vi "Main.vi"() -> ()   [LabVIEW 2019]
uses:
  SubVi/TypeDefs/ModeControl.ctl
  SubVi/TypeDefs/MotorDataControl.ctl
  SubVi/TypeDefs/PerturbationControl.ctl
  SubVi/TypeDefs/GameMode.ctl
  <vilib>/myRIO/Instrument Drivers/Onboard IO/AO/typedefs/AO Reference.ctl
  <vilib>/myRIO/Common/Instrument Driver Framework/Utilities/typedefs/myRIO Generic Hardware Reference.ctl
  <vilib>/myRIO/Common/Instrument Driver Framework/Utilities/typedefs/Hardware Version Enum.ctl
  <vilib>/myRIO/Common/Instrument Driver Framework/Utilities/typedefs/myRIO v1.0 Reference.ctl
  <vilib>/myRIO/Common/Instrument Driver Framework/Utilities/typedefs/Generic FPGA Reference.ctl
  <vilib>/myRIO/Common/Instrument Driver Framework/myRIO v1.0/AO/typedefs/AO Channels List.ctl
  <vilib>/myRIO/Common/Instrument Driver Framework/myRIO v1.0/AO/typedefs/AO Channels Enum.ctl
  <vilib>/myRIO/Common/Instrument Driver Framework/Utilities/typedefs/Analog Scaling Constants List.ctl
  <vilib>/myRIO/Common/Instrument Driver Framework/Utilities/typedefs/Analog Scaling Constants.ctl
  <vilib>/userDefined/High Color/nirio_resource_hc.ctl
  <vilib>/myRIO/Instrument Drivers/Onboard IO/DIO/typedefs/DIO Reference.ctl
  <vilib>/myRIO/Common/Instrument Driver Framework/myRIO v1.0/DIO/typedefs/DIO Channels List.ctl
  <vilib>/myRIO/Common/Instrument Driver Framework/myRIO v1.0/DIO/typedefs/DIO Channels Enum.ctl
  Tutorial/Shared VIs/TypeDef_TDMS_States.ctl
  <vilib>/Platform/TimedLoop/XDataNode/timing_clust.ctl
  <vilib>/Platform/TimedLoop/XDataNode/nitl_modes.ctl
  <vilib>/Platform/TimedLoop/XDataNode/wakeup.ctl
  SubVi/TypeDefs/PositionDataControl.ctl
  <vilib>/myRIO/Common/Instrument Driver Framework/myRIO v1.0/Encoder/typedefs/Encoder Signal Mode.ctl
  <vilib>/myRIO/Instrument Drivers/Onboard IO/Encoder/typedefs/Encoder Reference.ctl
  <vilib>/myRIO/Common/Instrument Driver Framework/myRIO v1.0/Encoder/typedefs/Encoder Channels Enum.ctl
  <vilib>/myRIO/Common/Instrument Driver Framework/myRIO v1.0/Encoder/typedefs/Encoder Configuration v1.0.ctl
  <vilib>/myRIO/Instrument Drivers/Onboard IO/AI/typedefs/AI Reference.ctl
  <vilib>/myRIO/Common/Instrument Driver Framework/myRIO v1.0/AI/typedefs/AI Channels List.ctl
  <vilib>/myRIO/Common/Instrument Driver Framework/myRIO v1.0/AI/typedefs/AI Channels Enum.ctl
  <vilib>/myRIO/Common/Instrument Driver Framework/Utilities/vis/Is FPGA Ref Available.vi
  <vilib>/myRIO/Common/Instrument Driver Framework/myRIO v1.0/AO/vis/myRIO v1.1 Open AO.vi
  <vilib>/myRIO/Instrument Drivers/Onboard IO/AO/vis/Write.vi
  <vilib>/myRIO/Common/Instrument Driver Framework/myRIO v1.0/DIO/vis/myRIO v1.1 Open DIO.vi
  <vilib>/myRIO/Instrument Drivers/Onboard IO/DIO/vis/Write.vi
  <vilib>/myRIO/Common/Instrument Driver Framework/myRIO v1.0/AI/vis/myRIO v1.1 Open AI.vi
  <vilib>/myRIO/Instrument Drivers/Onboard IO/AI/vis/Read.vi
  <vilib>/myRIO/Common/Instrument Driver Framework/myRIO v1.0/Encoder/vis/myRIO v1.1 Open Encoder.vi
  <vilib>/myRIO/Instrument Drivers/Onboard IO/Encoder/vis/Read.vi
  <vilib>/myRIO/Common/Instrument Driver Framework/Utilities/vis/Validate Channels.vi
  <vilib>/myRIO/Common/Instrument Driver Framework/myRIO v1.0/AO/vis/myRIO v1.0 Reserve AO.vi
  <vilib>/myRIO/Common/Instrument Driver Framework/myRIO v1.0/DIO/vis/myRIO v1.0 Reserve DIO.vi
  <vilib>/myRIO/Common/Instrument Driver Framework/myRIO v1.0/AI/vis/myRIO v1.0 Reserve AI.vi
  <vilib>/myRIO/Common/Instrument Driver Framework/myRIO v1.0/Encoder/vis/myRIO v1.0 Reserve Encoder.vi
  <vilib>/myRIO/Common/Instrument Driver Framework/myRIO v1.0/AO/vis/myRIO v1.0 Build MUX Configuration AO.vi
  <vilib>/myRIO/Common/Instrument Driver Framework/myRIO v1.0/Resource Manager/vis/myRIO v1.0 Reserve Channel List.vi
  <vilib>/myRIO/Common/Instrument Driver Framework/myRIO v1.0/DIO/vis/myRIO v1.0 Build MUX Configuration DIO.vi
  <vilib>/myRIO/Common/Instrument Driver Framework/myRIO v1.0/AI/vis/myRIO v1.0 Build MUX Configuration AI.vi
  <vilib>/myRIO/Common/Instrument Driver Framework/myRIO v1.0/Encoder/vis/myRIO v1.0 Build MUX Configuration Encoder.vi
  <vilib>/myRIO/Common/Instrument Driver Framework/myRIO v1.0/Resource Manager/vis/myRIO v1.0 Reserve Channel.vi
  <vilib>/myRIO/Common/Instrument Driver Framework/myRIO v1.0/Resource Manager/vis/myRIO v1.0 Unreserve Channel.vi
  <vilib>/myRIO/Common/Instrument Driver Framework/myRIO v1.0/Resource Manager/vis/myRIO v1.0 Create Configuration List.vi
  <vilib>/myRIO/Common/Instrument Driver Framework/myRIO v1.0/Resource Manager/vis/myRIO v1.0 Build Mutex Name.vi
  <vilib>/Utility/VariantDataType/GetNumericInfo.vi
  <vilib>/Utility/error.llb/Error Cluster From Error Code.vi
  <vilib>/myRIO/Common/Instrument Driver Framework/myRIO v1.0/myRIO v1.1 Open.vi
  <vilib>/myRIO/Common/Instrument Driver Framework/myRIO v1.0/AO/vis/myRIO v1.0 Get Scaling Constants AO.vi
  <vilib>/myRIO/Common/Instrument Driver Framework/Utilities/vis/IO Manager.vi
  <vilib>/myRIO/Common/Instrument Driver Framework/Utilities/vis/Configuration Manager.vi
  <vilib>/myRIO/Common/Instrument Driver Framework/myRIO v1.0/myRIO v1.0 Close.vi
  <vilib>/myRIO/Common/Instrument Driver Framework/myRIO v1.0/AO/vis/myRIO v1.0 Write AO.vi
  <vilib>/myRIO/Common/Instrument Driver Framework/myRIO v1.0/Resource Manager/vis/myRIO v1.0 Configure IO.vi
  <vilib>/myRIO/Common/Instrument Driver Framework/myRIO v1.0/DIO/vis/myRIO v1.0 Write DIO.vi
  <vilib>/myRIO/Common/Instrument Driver Framework/myRIO v1.0/Encoder/vis/myRIO v1.0 Configure Encoder.vi
  <vilib>/myRIO/Common/Instrument Driver Framework/myRIO v1.0/Encoder/vis/myRIO v1.0 Read Encoder.vi
  <vilib>/myRIO/Common/Instrument Driver Framework/myRIO v1.0/AI/vis/myRIO v1.0 Get Scaling Constants AI.vi
  <vilib>/myRIO/Common/Instrument Driver Framework/myRIO v1.0/AI/vis/myRIO v1.0 Read AI.vi
  <vilib>/addons/control/pid/pid.llb/PID (DBL).vi
  <vilib>/myRIO/Express VI/Onboard IO/AO/AO Express VI.xnode
  <vilib>/myRIO/Instrument Drivers/Onboard IO/AO/vis/myRIO AO Open.xnode
  <vilib>/myRIO/Express VI/Onboard IO/DO/DO Express VI.xnode
  <vilib>/myRIO/Instrument Drivers/Onboard IO/DIO/vis/myRIO DIO Open.xnode
  <vilib>/Platform/TimedLoop/XDataNode/XDataNode.xnode
  <vilib>/myRIO/Express VI/Onboard IO/Encoder/Encoder Express VI.xnode
  <vilib>/myRIO/Instrument Drivers/Onboard IO/Encoder/vis/myRIO Encoder Open.xnode
  <vilib>/myRIO/Common/Instrument Driver Framework/myRIO v1.0/Encoder/typedefs/Encoder Count Direction Enum.ctl
  <vilib>/myRIO/Express VI/Onboard IO/AI/AI Express VI.xnode
  <vilib>/myRIO/Instrument Drivers/Onboard IO/AI/vis/myRIO AI Open.xnode
  <vilib>/Platform/TimedLoop/XDataNode/XDNodeRunTimeDep.lvlib
  <vilib>/addons/control/pid/NI_PID_pid.lvlib
  <vilib>/myRIO/Instrument Drivers/Onboard IO/AO/AO.lvlib
  <vilib>/myRIO/Instrument Drivers/Onboard IO/DIO/DIO.lvlib
  <vilib>/myRIO/Instrument Drivers/Onboard IO/Encoder/Encoder.lvlib
  <vilib>/myRIO/Instrument Drivers/Onboard IO/AI/AI.lvlib
panel:
  out "LinPot mm (center to finger) 2":dbl
  out "LinPot mm (center to finger)":dbl
  out "Right Poti Offset":dbl
  out "Left Poti Offset":dbl
  out "Right Poti Gradient":dbl
  out "Left Poti Gradient":dbl
  out "LX gradient":dbl
  out "LY gradient":dbl
  out "RY gradient":dbl
  out "RX gradient":dbl
  out "Safety Warning":bool
  out "Safety Been Triggered":bool
  out "TimeStampData":cluster{"time":string}
  out "UDPTimestamp":T1
  out "Force Sensor Faulty":bool
  out "Pots Faulty":bool
  out "ForceBiasGR_R":dbl
  out "ForceBiasPS_R":dbl
  out "Left F_y[N]":dbl(graph)
  out "Left F_x[N]":dbl(graph)
  out "define_dX_GR":bool
  out "Applied Torque Rotation":dbl(graph)
  out "PS Setpoint/ProcessVar [mm]":T2(graph) caption="Response"
  out "dtheta PS (deg)":dbl
  out "GR Setpoint/ProcessVar [mm]":T2(graph) caption="Response"
  out "dx GR (mm)":dbl
  out "Potentiometers_array":dbl[](array[numeric])
  out "PID output voltage rotation":dbl(graph)
  out "PID output voltage translation":dbl(graph)
  out "ForceBiasGR_L":dbl
  out "ForceBiasPS_L":dbl
  out "NewPerturbation":bool
  out "JSON string":string
  out "Baseline[N]":dbl
  out "Reached":bool
  out "ForcePeak[N]":dbl
  out "ForceTransBuffer[N]":ext[](array[numeric])
  out "Game":T4
  out "UDPPerturbation":T5
  out "Perturbation":T6
  out "MotorData":T7
  out "UDPGame":T5
  in  "SaveData (Manual)":bool
  out "Main Loop Time":i32
  out "Perturbation Response":cluster{"PositionTranslation":dbl, "Step":dbl}(graph) caption="Response"
  out "Target Position Rotation":dbl format="%#_13g"
  out "Target Position Translation":dbl format="%#_13g"
  out "Relative Pos Trans Saved":dbl format="%#_13g"
  out "Save Data":bool=TRUE
  out "isaved":i32
  out "Case":i32
  out "UDPSafety":T5
  out "InitialTranslation":dbl
  out "InitialRotation":dbl
  out "HardSafety":bool
  out "SoftSafety":bool
  out "AppliedTorqueRotation [Nmm]":dbl
  out "AbsolutePositionRotation":dbl
  out "AbsolutePositionTranslation":dbl
  out "AppliedForceRotation [N]":dbl
  out "AppliedForceTranslation [N]":dbl
  out "Right F_y[N]":dbl(graph)
  out "Right F_x[N]":dbl(graph)
  out "Finalize":bool
  out "VoltageTranslation":dbl
  out "VoltageRotation":dbl
  out "Calibration":T8
  out "Mode":T9
  out "MotorValues":T10
  out "UDPMotorValues":T5
  out "VelocityRotation":dbl
  out "VelocityTranslation":dbl
  out "CalibratorTranslation":dbl
  out "CalibratorRotation":dbl
  out "Period":i32
  out "LoopTime":dbl
  out "RelativePositionRotation":dbl
  out "RelativePositionTranslation":dbl
  out "UDPCalibration":T5
  out "UDPMotorData":T5
  out "UDPMode":T5
  out "IPAddress":i64
  out "UDPConnection":T5
  # "HELLO UPDATE"
  # "Green if data saving in progress"
  # "Force manual data save when pressed"
  # "To Giorgia:\nremember first to set \nthis index to 0 if you\nwant to control the\npronosupination DOF\nor to 1 if you want to\ncontrol the grasping\n\nAlways remember \nto set the stopPosition\n(for stop mode), \nor position&velocity (for\nmove mode) in a way that\nis feasible for the \nRelativePosition in which\nyou are. Do that ALWAYS \n1) before changing motorMode\n2) before changing \nMode from Wait to Run"
  # "Perturbation response in grasping"
  # "Green ON = no safety stop\nSoft = max force/pos/vel exceeded\nHard= sensor problem"
  # "Green ON = closing Labview \n(on Hard Safety or\nquit GUI/patient selection)"
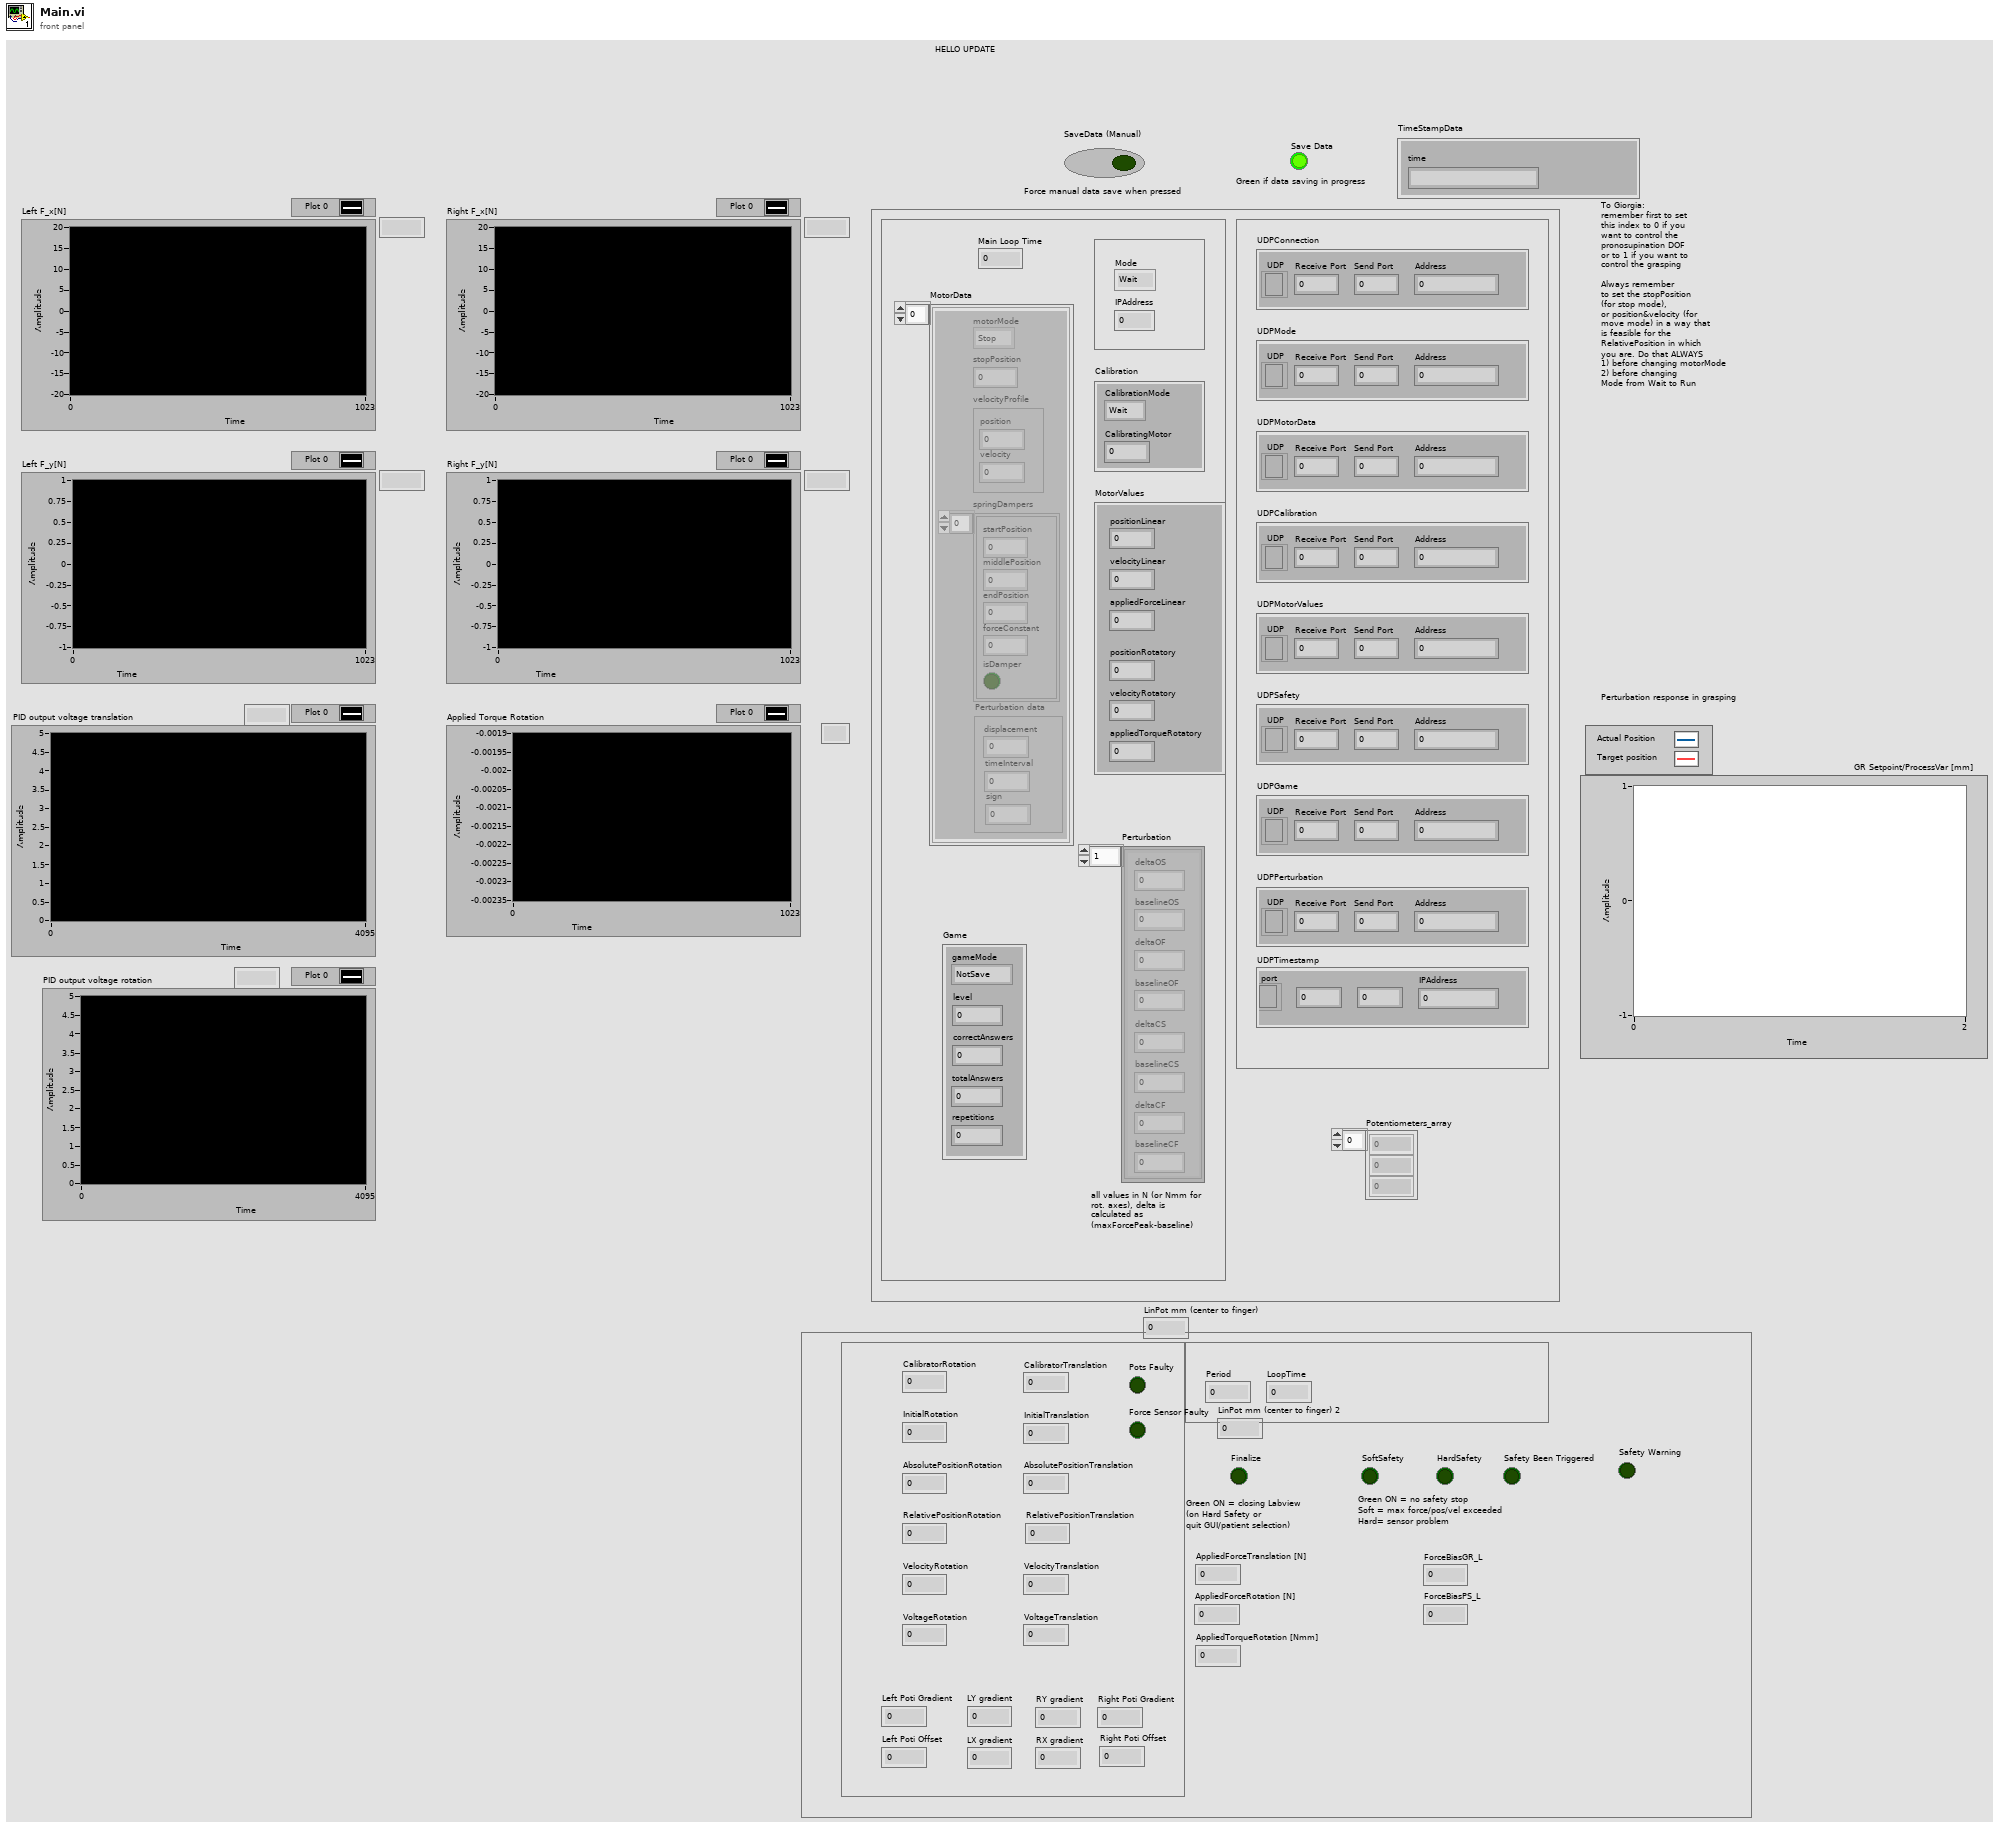
[diagram p1: front panel]
types:
  T1 = cluster{"port":refnum<k16>, i32, i32, "IPAddress":i64}
  T2 = cluster{"AbsolutePositionTranslation":dbl, "inverse delta GR":dbl}
  T3 = typedef "GameMode.ctl" = enum16{"NotSave", "Calibrate", "Training", "Test", "Summary"}
  T4 = cluster{"gameMode":T3, "level":dbl, "correctAnswers":dbl, "totalAnswers":dbl, "repetitions":dbl}
  T5 = cluster{"UDP":refnum<k16>, "Receive Port":i32, "Send Port":i32, "Address":i64}
  T6 = typedef "PerturbationControl.ctl" = cluster{"deltaOS":dbl, "baselineOS":dbl, "deltaOF":dbl, "baselineOF":dbl, "deltaCS":dbl, "baselineCS":dbl, "deltaCF":dbl, "baselineCF":dbl}[]
  T7 = typedef "MotorDataControl.ctl" = cluster{"motorMode":enum16{"Stop", "Move", "Force", "Perturbation"}, "stopPosition":dbl, "velocityProfile":cluster{"position":dbl, "velocity":dbl}, "springDampers":cluster{"startPosition":dbl, "middlePosition":dbl, "endPosition":dbl, "forceConstant":dbl, "isDamper":bool}[], "Perturbation data ":cluster{"displacement":dbl, "timeInterval":dbl, "sign":i64}}[]
  T8 = cluster{"CalibrationMode":enum16{"Wait", "Calibrate"}, "CalibratingMotor":i8}
  T9 = typedef "ModeControl.ctl" = enum16{"Wait", "Calibrate", "Run", "Safety", "Quit"}
  T10 = cluster{"positionLinear":dbl, "velocityLinear":dbl, "appliedForceLinear":dbl, "positionRotatory":dbl, "velocityRotatory":dbl, "appliedTorqueRotatory":dbl}
  T11 = typedef "AO.lvlib/AO Reference.ctl" = cluster{"myRIO Reference":T12, "AO Channel List":T16, "AO Scaling Constant List":T18}
  T12 = typedef "myRIO Generic Hardware Reference.ctl" = cluster{"myRIO Model":T13, "myRIO Hardware Reference":T14}
  T13 = typedef "Hardware Version Enum.ctl" = enum16{"Unknown", "myRIO-1900", "myRIO-1950", "roboRIO", "NI ELVIS RIO CM", "ELVIS III"}
  T14 = typedef "myRIO v1.0 Reference.ctl" = cluster{"Generic FPGA Reference":T15, "Allow multiple opens":bool}
  T15 = typedef "Generic FPGA Reference.ctl" = refnum<k20>
  T16 = typedef "AO Channels List.ctl" = T17[]
  T17 = typedef "AO Channels Enum.ctl" = enum16{"Not Connected", "AudioOut/Left", "AudioOut/Right", "C/AO0", "C/AO1", "A/AO0", "A/AO1", "B/AO0", "B/AO1"}
  T18 = typedef "Analog Scaling Constants List.ctl" = T19[]
  T19 = typedef "Analog Scaling Constants.ctl" = cluster{"LSB Weight (Volts)":dbl, "Offset (Volts)":dbl, "Signed?":bool}
  T20 = typedef "nirio_resource_hc.ctl" = tag
  T21 = typedef "DIO.lvlib/DIO Reference.ctl" = cluster{"myRIO Reference":T12, "DIO Channels List":T22}
  T22 = typedef "DIO Channels List.ctl" = T23[]
  T23 = typedef "DIO Channels Enum.ctl" = enum16{"Not Connected", "C/DIO0", "C/DIO1", "C/DIO2", "C/DIO3", "C/DIO4", "C/DIO5", "C/DIO6", "C/DIO7", "A/DIO0", "A/DIO1", "A/DIO2", "A/DIO3", "A/DIO4", "A/DIO5", "A/DIO6", "A/DIO7", "A/DIO8", "A/DIO9", "A/DIO10", "A/DIO11", "A/DIO12", "A/DIO13", "A/DIO14", "A/DIO15", "A/DIO16", "A/DIO17", "A/DIO18", "A/DIO19", "B/DIO0", "B/DIO1", "B/DIO2", "B/DIO3", "B/DIO4", "B/DIO5", "B/DIO6", "B/DIO7", "B/DIO8", "B/DIO9", "B/DIO10", "B/DIO11", "B/DIO12", "B/DIO13", "B/DIO14", "B/DIO15", "B/DIO16", "B/DIO17", "B/DIO18", "B/DIO19", "LED0", "LED1", "LED2", "LED3", "Button0", "DIO/DIO0", "DIO/DIO1", "DIO/DIO2", "DIO/DIO3", "DIO/DIO4", "DIO/DIO5", "DIO/DIO6", "DIO/DIO7", "DIO/DIO8", "DIO/DIO9", "SPI/CS0", "SPI/CS1", "SPI/CS2", "SPI/CS3", "LED RADIO (Green)", "LED RADIO (Red)", "LED COMM (Green)", "LED COMM (Red)", "LED MODE (Green)", "LED MODE (Red)"}
  T24 = typedef "TypeDef_TDMS_States.ctl" = enum16{"Do Nothing", "Create", "Write", "Close"}
  T25 = enum16{"open", "open or create", "create or replace", "create", "open (read-only)"}
  T26 = typedef "XDNodeRunTimeDep.lvlib/timing_clust.ctl" = cluster{"Expected End [f-1]":u64, "Actual End [f-1]":u64, "Finished Late? [f-1]":bool, "Expected End [i-1]":u64, "Actual End [i-1]":u64, "Finished Late? [i-1]":bool, "Expected Start [i]":u64, "Actual Start [i]":u64, "Expected Start [f]":u64, "Actual Start [f]":u64, "Source Name":string, "Structure Name":string, "Period":i64, "Deadline":i64, "Offset":i64, "Start":i64, "Priority":i32, "Timeout":i32, "Mode":T27, "Wakeup Reason":T28, "Error":errorcluster, "Source Type":string, "Secondary Source Type":string, "Global End Time":u64, "Global Start Time":u64, "Frame Duration":u64, "Iteration Duration":u64, "Assigned CPU":i32, "I/O Scan Engine Mode":u32}
  T27 = typedef "XDNodeRunTimeDep.lvlib/nitl_modes.ctl" = enum32{"No Change", "Process missed periods, maintain original phase", "Discard missed periods, maintain original phase", "Process missed periods, ignore original phase", "Discard missed periods, ignore original phase"}
  T28 = typedef "XDNodeRunTimeDep.lvlib/wakeup.ctl" = enum32{"Normal", "Aborted", "Asynchronous wakeup", "Timing source error", "Timed loop error", "Timeout"}
  T29 = typedef "PositionDataControl.ctl" = cluster{"Position":dbl, "Velocity":dbl}
  T30 = typedef "AI.lvlib/AI Reference.ctl" = cluster{"myRIO Reference":T12, "AI Channels List":T31, "AI Scaling Constants List":T18}
  T31 = typedef "AI Channels List.ctl" = T32[]
  T32 = typedef "AI Channels Enum.ctl" = enum16{"Not Connected", "AudioIn/Left", "AudioIn/Right", "C/AI0", "C/AI1", "A/AI0", "A/AI1", "A/AI2", "A/AI3", "A/AI4", "A/AI5", "A/AI6", "A/AI7", "B/AI0", "B/AI1", "B/AI2", "B/AI3", "B/AI4", "B/AI5", "B/AI6", "B/AI7", "AI/AI0", "AI/AI1", "AI/AI2", "AI/AI3", "A/AI0 (DIFF)", "A/AI1 (DIFF)", "A/AI2 (DIFF)", "A/AI3 (DIFF)", "B/AI0 (DIFF)", "B/AI1 (DIFF)", "B/AI2 (DIFF)", "B/AI3 (DIFF)"}
  T33 = typedef "Encoder.lvlib/Encoder Reference.ctl" = cluster{"myRIO Reference":T12, "Encoder Channels Enum":T34}
  T34 = typedef "Encoder Channels Enum.ctl" = enum16{"Not Connected", "C/ENC0", "C/ENC1", "A/ENC", "A/ENC0", "A/ENC1", "A/ENC2", "A/ENC3", "A/ENC4", "A/ENC5", "A/ENC6", "A/ENC7", "A/ENC8", "A/ENC9", "B/ENC", "B/ENC0", "B/ENC1", "B/ENC2", "B/ENC3", "B/ENC4", "B/ENC5", "B/ENC6", "B/ENC7", "B/ENC8", "B/ENC9", "DIO/ENC0", "DIO/ENC1", "DIO/ENC2", "DIO/ENC3", "DIO/ENC4"}
  T35 = typedef "Encoder Signal Mode.ctl" = enum16{"Quadrature phase signal", "Step and direction signal"}
  T36 = cluster{"startPosition":dbl, "middlePosition":dbl, "endPosition":dbl, "forceConstant":dbl, "isDamper":bool}[]
  T37 = cluster{"proportional gain (Kc)":dbl, "integral time (Ti, min)":dbl, "derivative time (Td, min)":dbl}
  T38 = cluster{"motorMode":enum16{"Stop", "Move", "Force", "Perturbation"}, "stopPosition":dbl, "velocityProfile":cluster{"position":dbl, "velocity":dbl}, "springDampers":cluster{"startPosition":dbl, "middlePosition":dbl, "endPosition":dbl, "forceConstant":dbl, "isDamper":bool}[], "Perturbation data ":cluster{"displacement":dbl, "timeInterval":dbl, "sign":i64}}
  T39 = cluster{"deltaOS":dbl, "baselineOS":dbl, "deltaOF":dbl, "baselineOF":dbl, "deltaCS":dbl, "baselineCS":dbl, "deltaCF":dbl, "baselineCF":dbl}
  T40 = cluster{"motorMode":enum16{"Stop", "Move", "Force", "Perturbation"}, "stopPosition":dbl, "velocityProfile":cluster{"position":dbl, "velocity":dbl}, "springDampers":cluster{"startPosition":dbl, "middlePosition":dbl, "endPosition":dbl, "forceConstant":dbl, "isDamper":bool}[], "Perturbation data ":cluster{"displacement":dbl, "timeInterval":dbl, "sign":i64}}[]
  T41 = cluster{"deltaOS":dbl, "baselineOS":dbl, "deltaOF":dbl, "baselineOF":dbl, "deltaCS":dbl, "baselineCS":dbl, "deltaCF":dbl, "baselineCF":dbl}[]
  T42 = cluster{"displacement":dbl, "timeInterval":dbl, "sign":i64}
  T43 = cluster{"RelativePositionTranslation":dbl, "dx GR (mm)":dbl}
  T44 = cluster{"RelativePositionTranslation":dbl, "RelativePositionTranslation":dbl}
  T45 = cluster{"RelativePositionRotation":dbl, "dtheta PS (deg)":dbl}
  T46 = cluster{"gameMode":i8, "level":dbl, "correctAnswers":dbl, "totalAnswers":dbl, "repetitions":dbl}
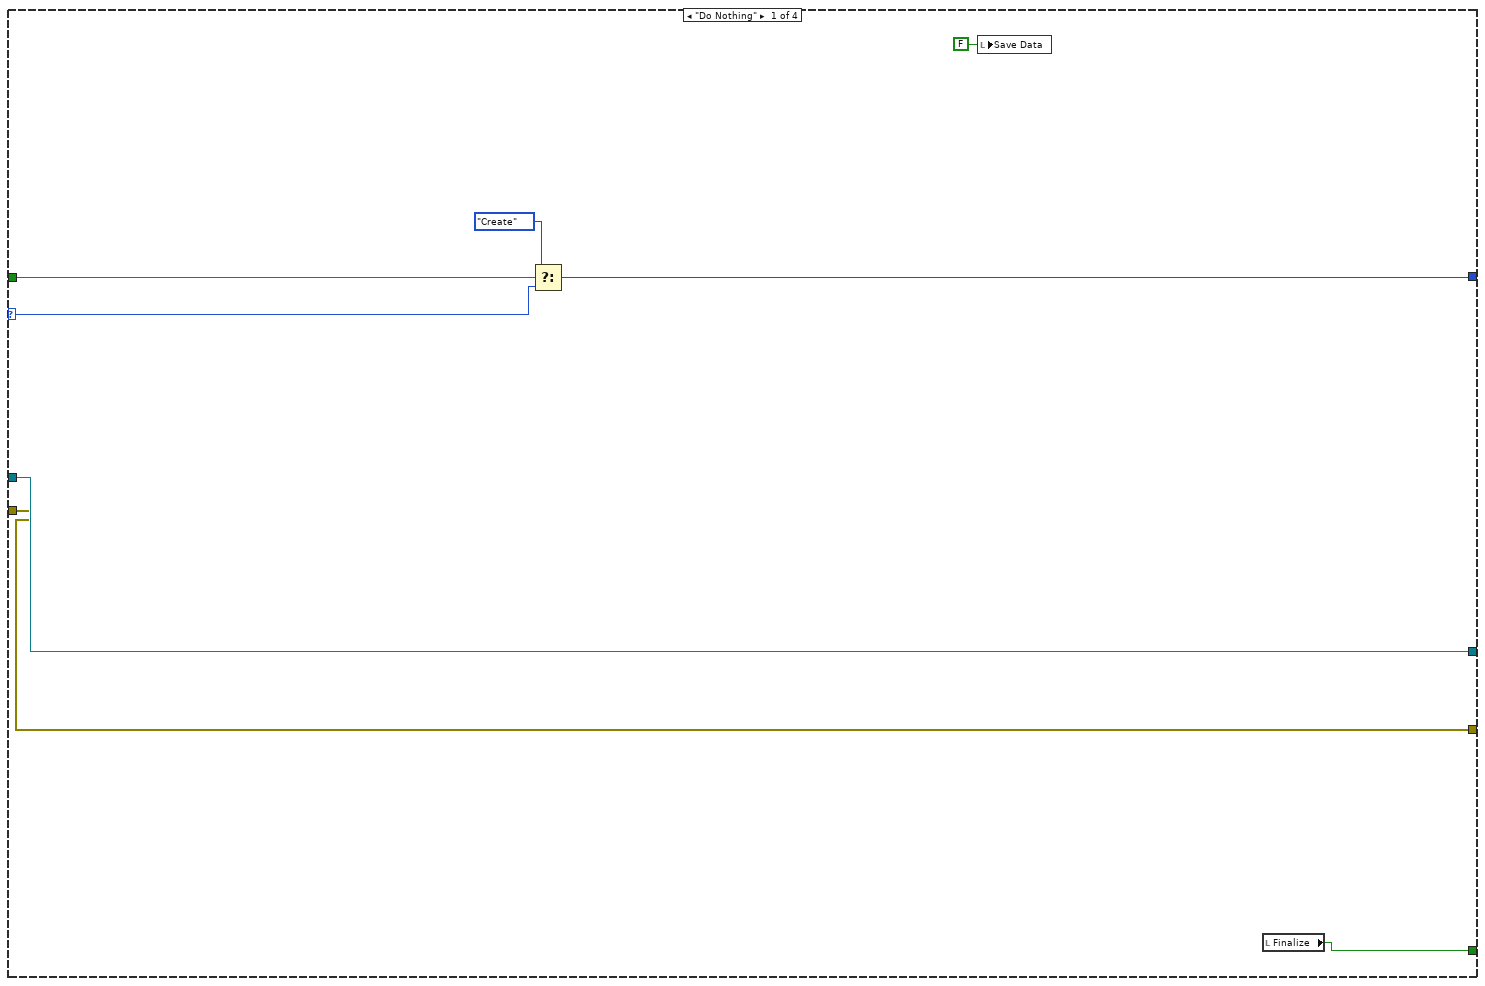
[diagram p2: hidden frame]
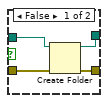
[diagram p3: hidden frame]
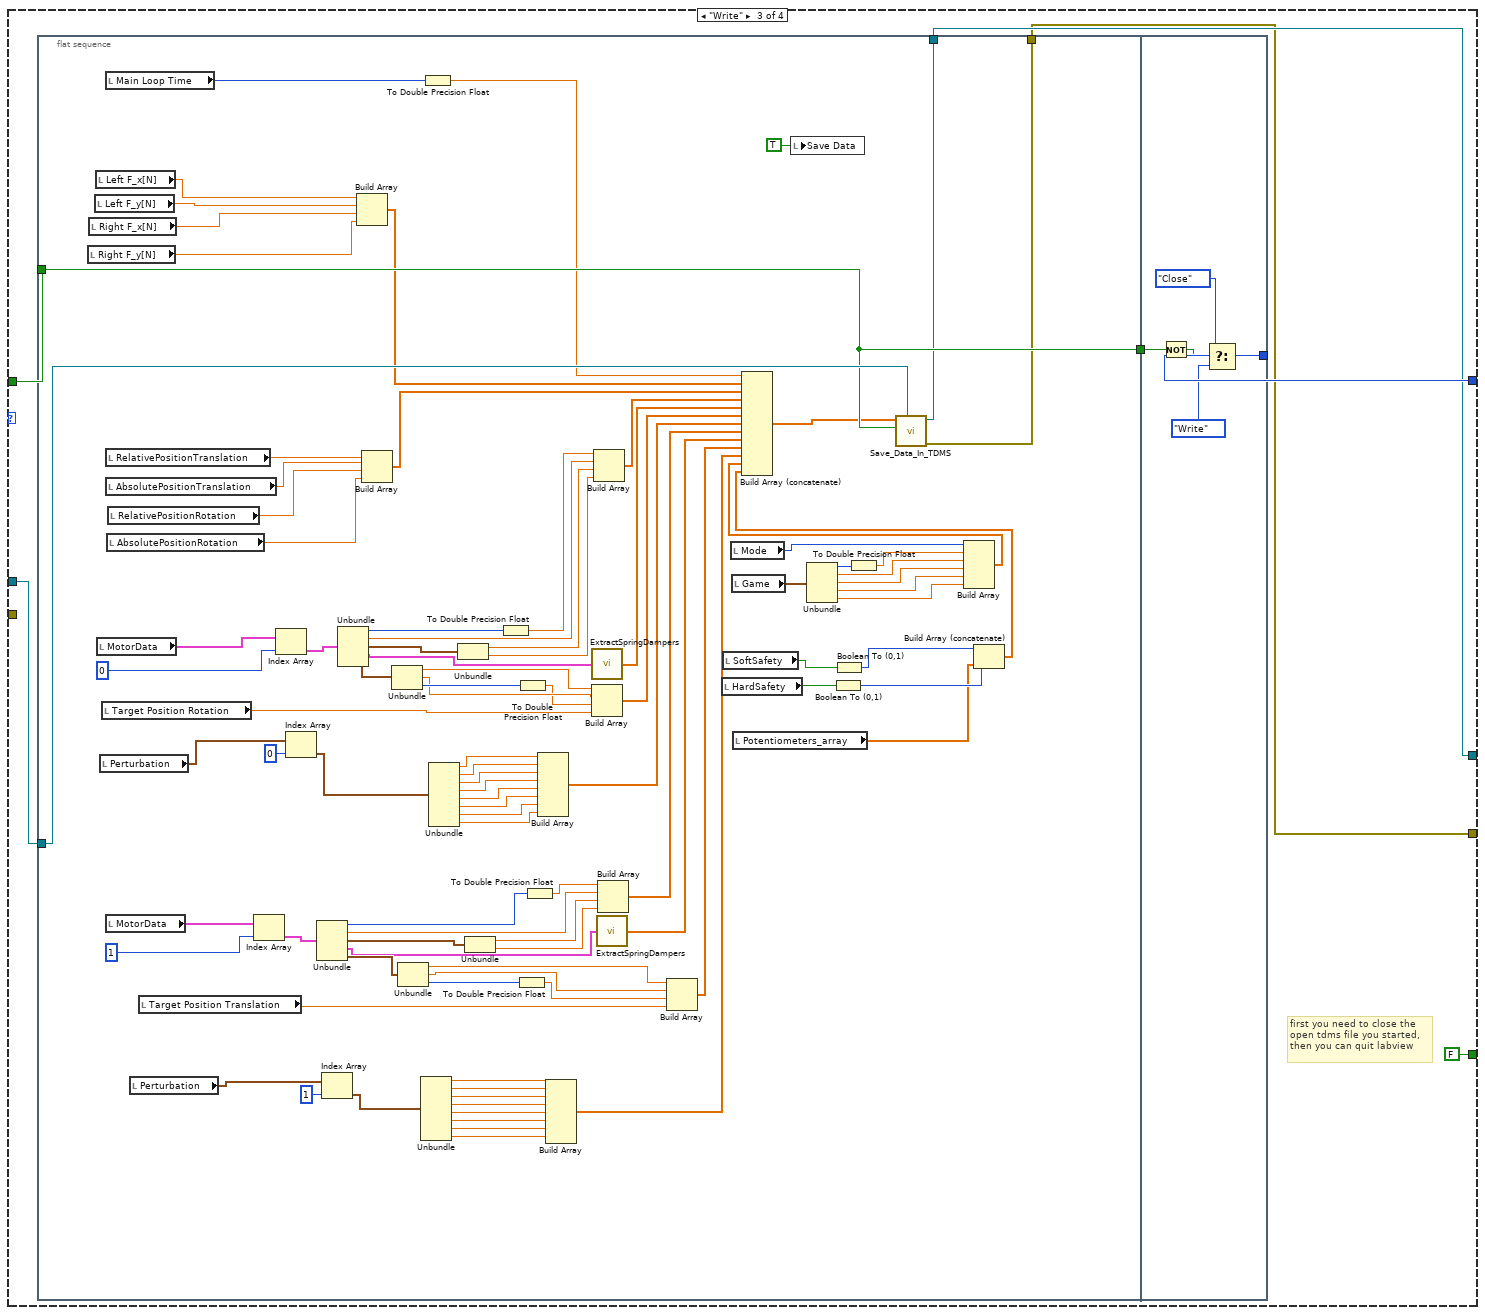
[diagram p4: hidden frame]
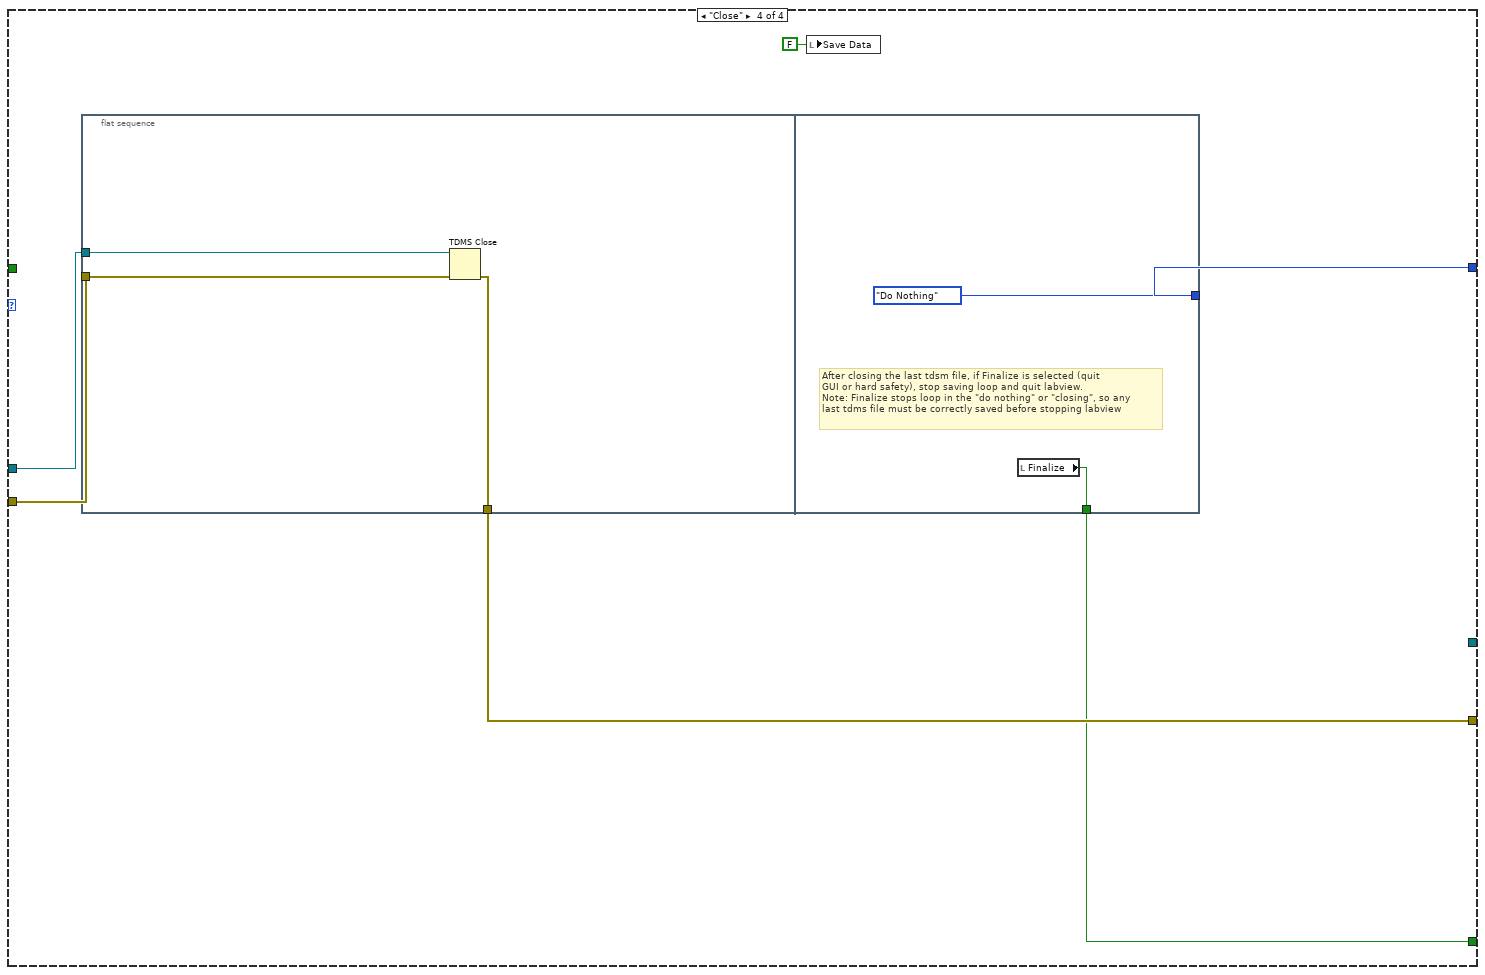
[diagram p5: hidden frame]
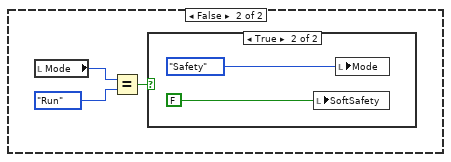
[diagram p8: hidden frame]
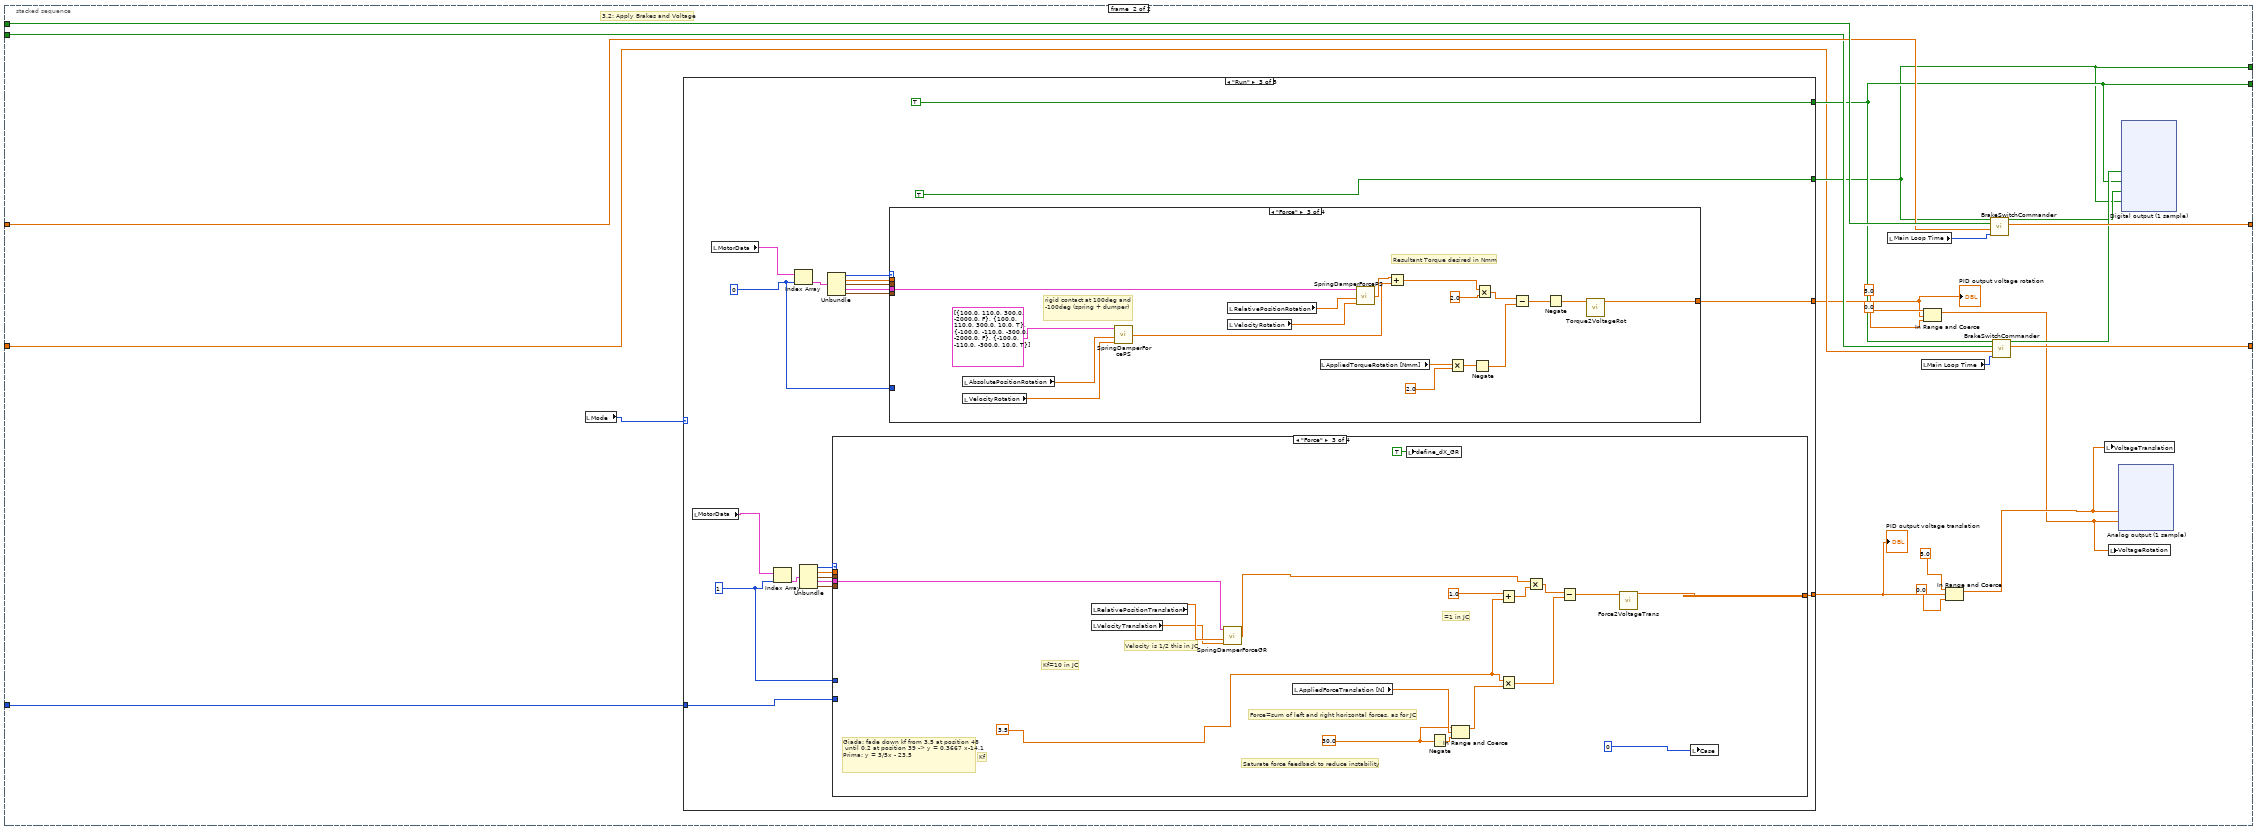
[diagram p10: hidden frame]
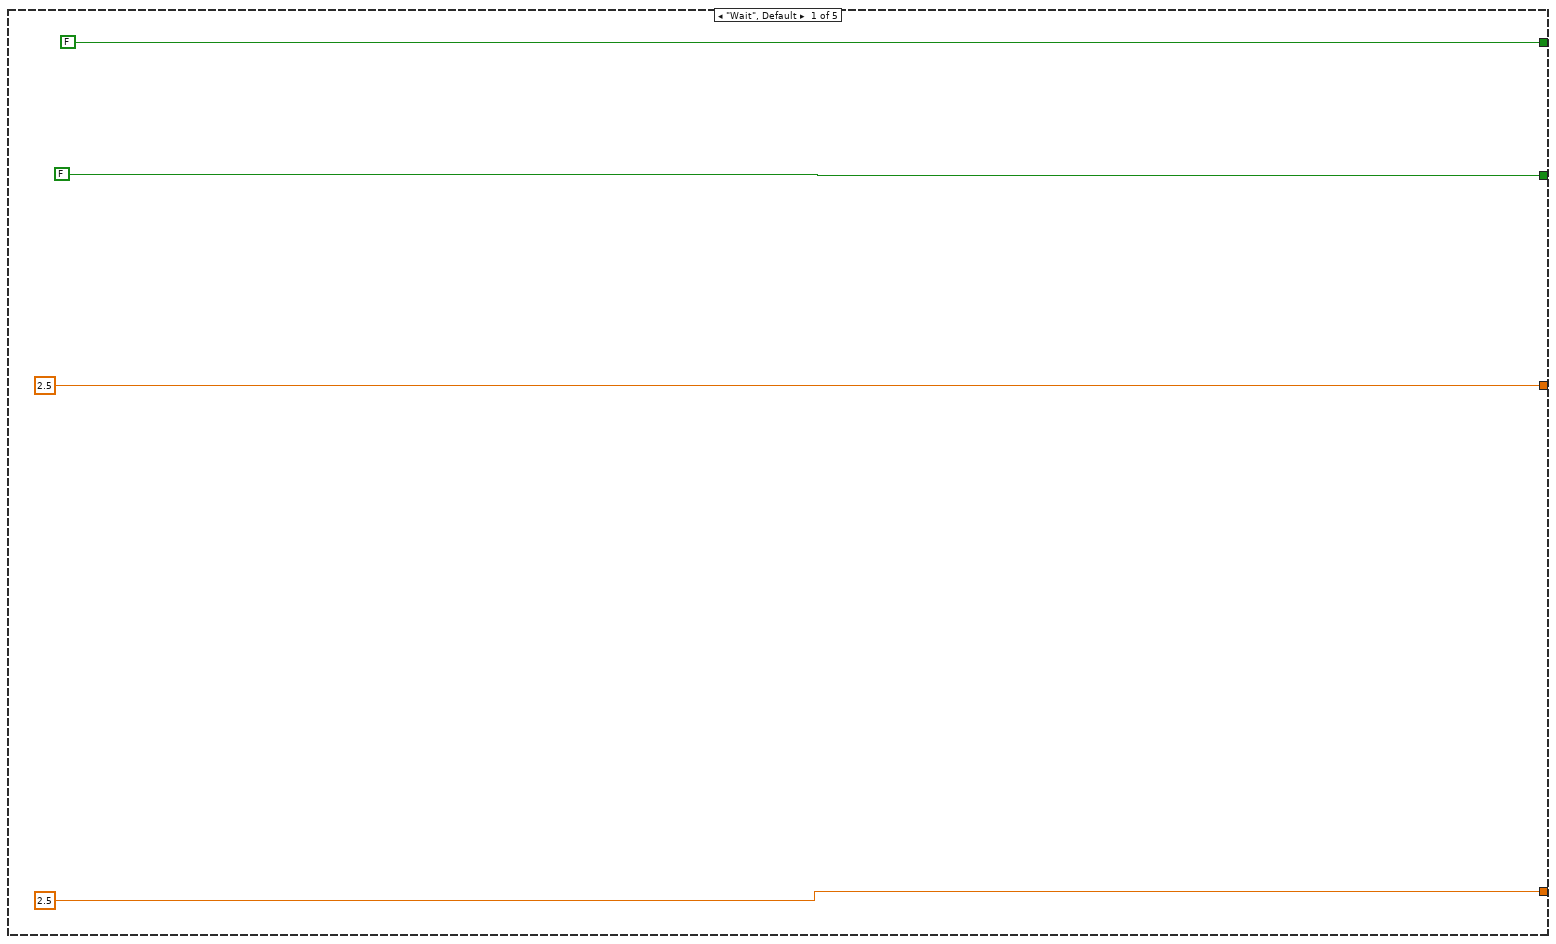
[diagram p11: hidden frame]
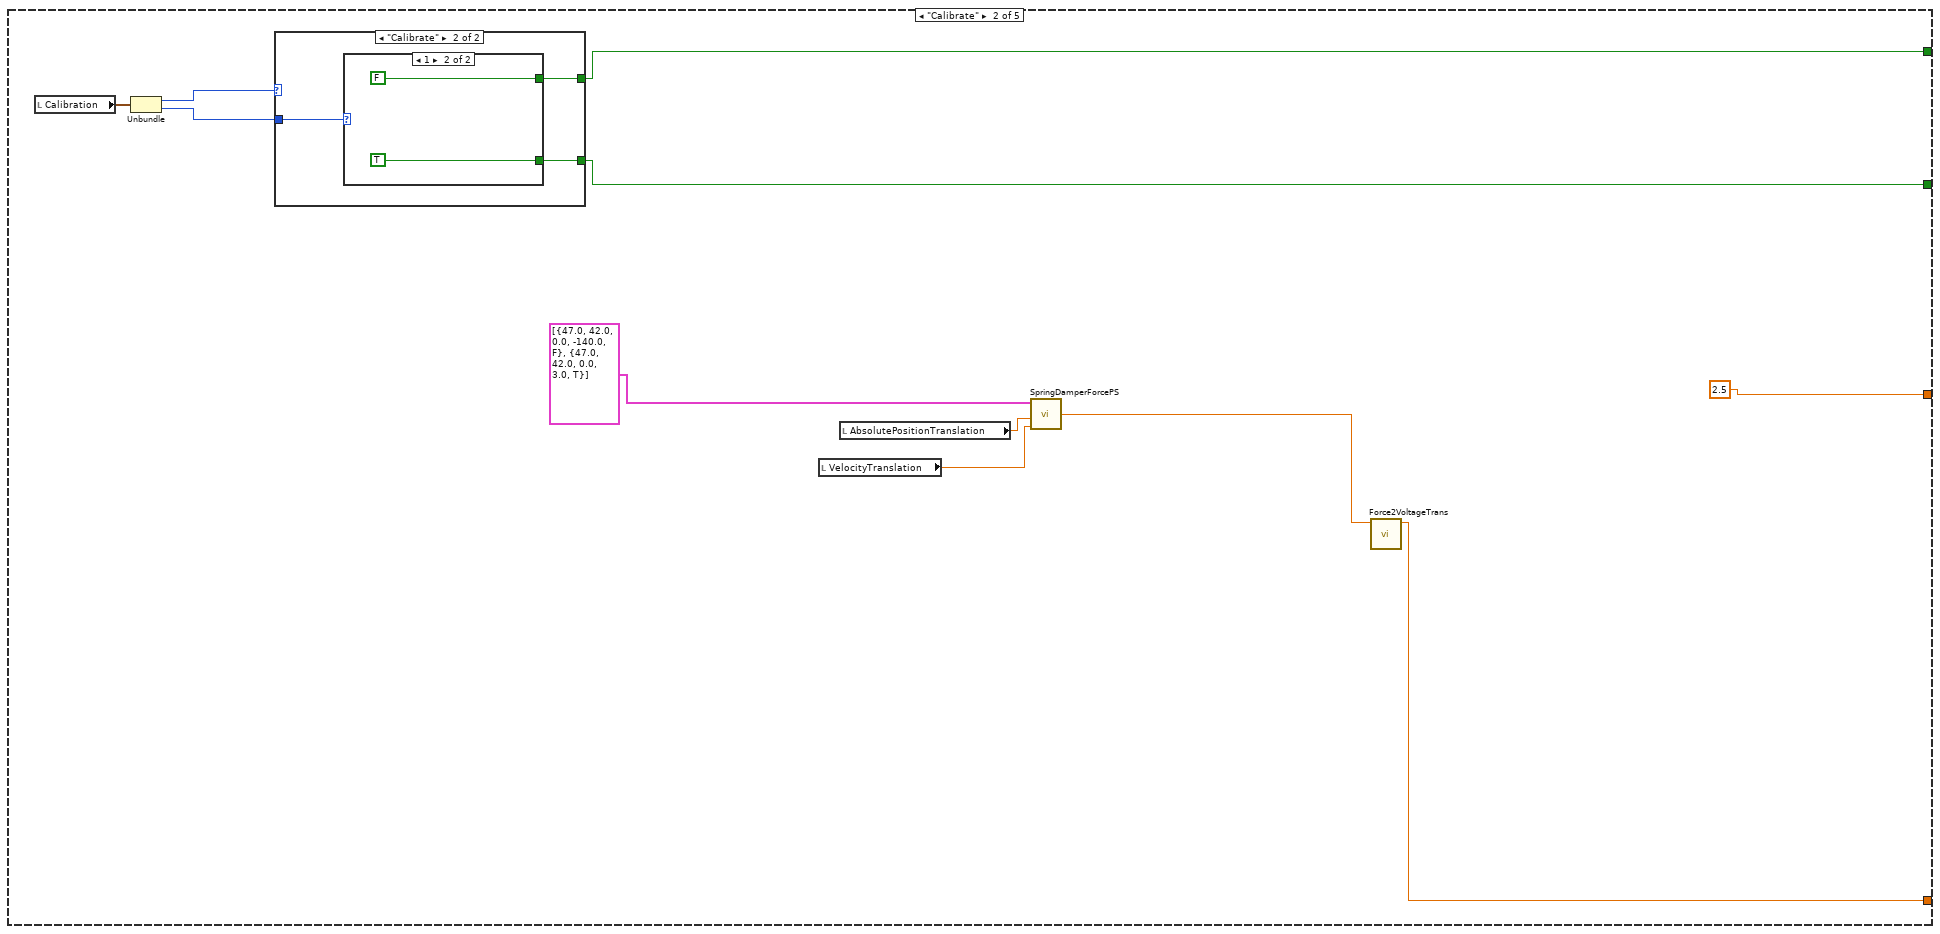
[diagram p12: hidden frame]
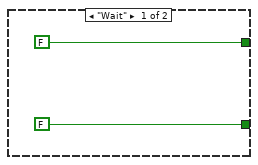
[diagram p13: hidden frame]
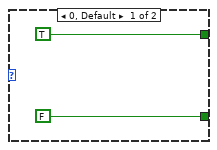
[diagram p14: hidden frame]
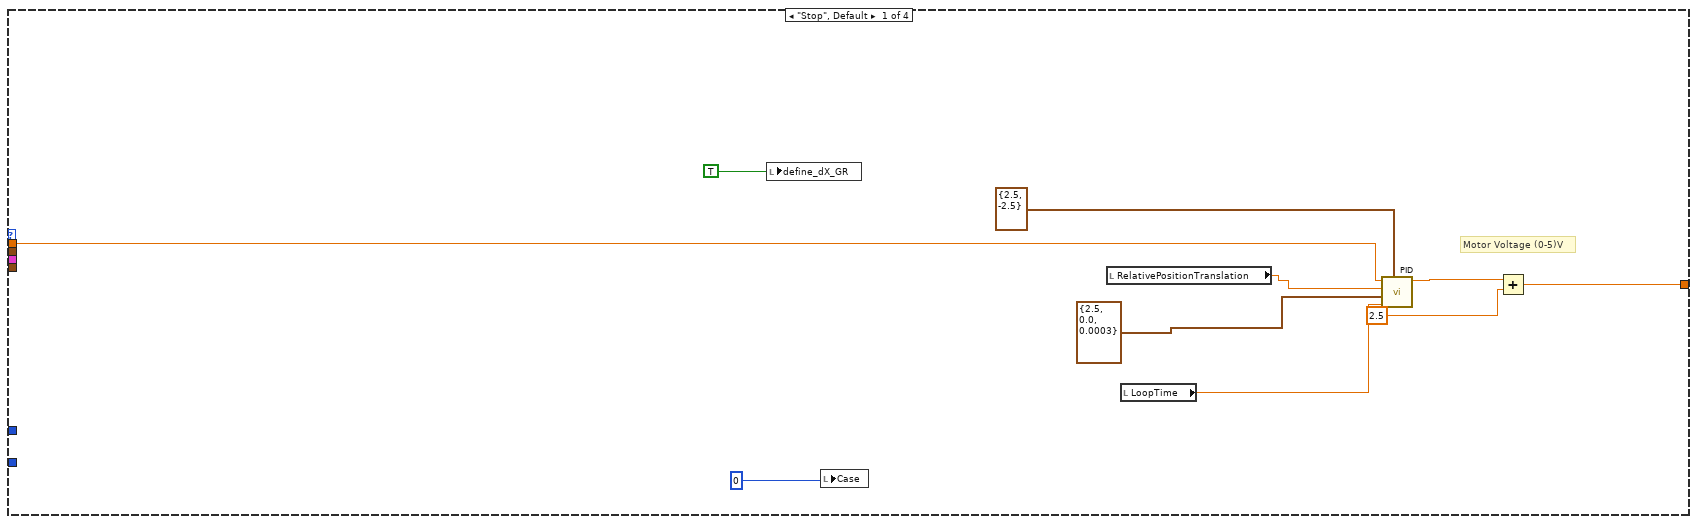
[diagram p15: hidden frame]
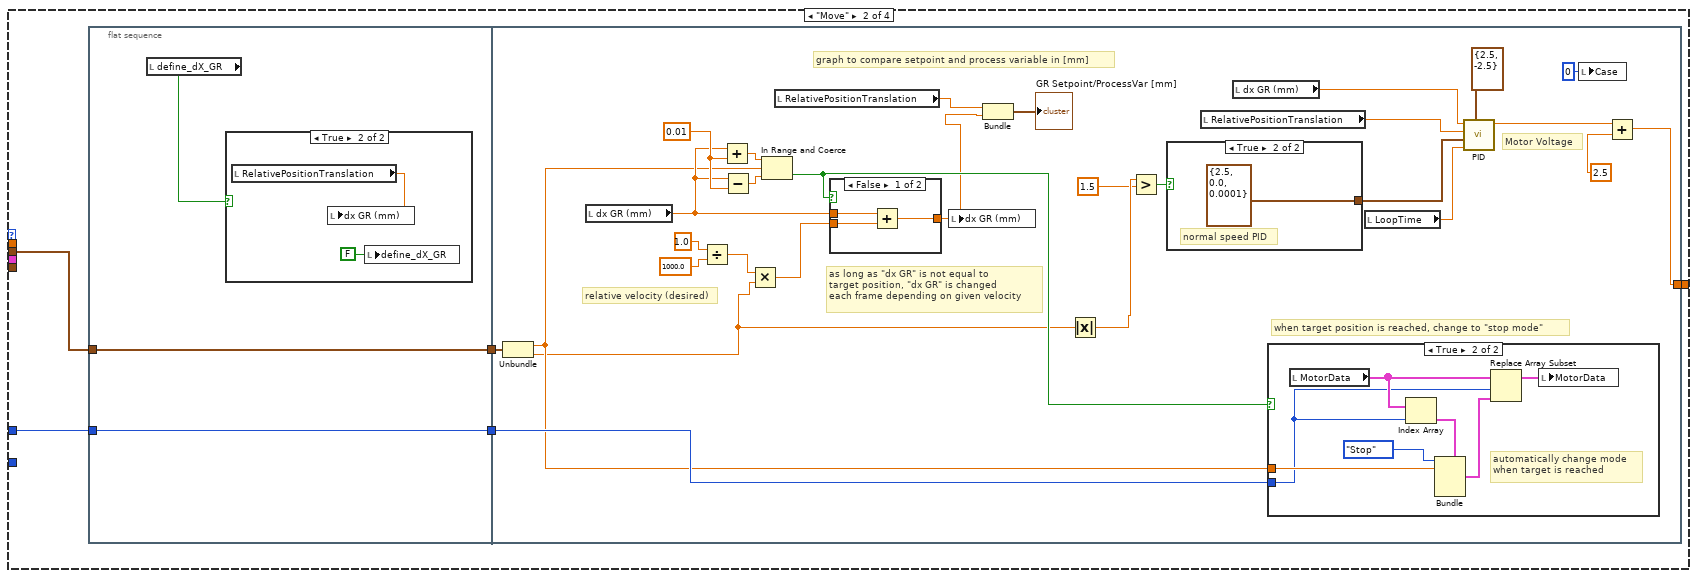
[diagram p16: hidden frame]
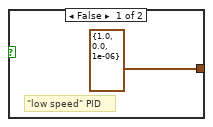
[diagram p18: hidden frame]
diagram:
  n1 = flat-sequence {
    frame #0 {
      w25 = 1000
      w45 = "172.22.11.1"  # address
      # "intermediate variables used within the calibration mode"
      # "intermediate variables used within the perturbation mode"
      # "RR 29.11.2019: Use IP\"255.255.255.255\" to find any device\nwhen Unity scripts are in \"Ethernet mode\"\nRR 09.02.2021: use IP 172.22.11.1 to use Unity scripts in \n\"HandyBot\" mode"
      # "0: Initialize Variables"
      n2 = local read "MotorData"() -> (w24:T7)
      n3 = call "ReadParams.vi"() -> ("Force RY"=→"RY gradient":dbl, "Force RX"=→"RX gradient":dbl, "Force LY"=→"LY gradient":dbl, "Force LX"=→"LX gradient":dbl, "Left Pot Gradient"=→"Left Poti Gradient":dbl, "Right Pot Offset"=→"Right Poti Offset":dbl, "Left Pot Offset"=→"Left Poti Offset":dbl, "Right Pot Gradient"=→"Right Poti Gradient":dbl)  [unwired: 4 in]
      n4 = local read "Perturbation"() -> (w19:T6)
      n5 = To Double Precision Float(number=w25) -> (double precision float=w43:dbl)
      n6 = Index Array(array=w24, index=0) -> (element=w35:T38)
      n7 = Index Array(array=w19, index=0) -> (element=w21:T39)
      n8 = Reciprocal(x=w43) -> (1/x=→"LoopTime":dbl)
      n9 = String To IP(1:w45) -> (0:→"IPAddress":u32)
      n10 = Initialize Array(w35, 2) -> (→"MotorData":T40)
      n11 = Initialize Array(w21, 2) -> (→"Perturbation":T41)
      "Period" <- w25
      "RelativePositionRotation" <- 0.0
      "RelativePositionTranslation" <- 0.0
      "VelocityTranslation" <- 0.0
      "VelocityRotation" <- 0.0
      "Mode" <- ModeControl."Wait" ("Mode")
      "Finalize" <- FALSE ("Finalize")
      "AppliedForceTranslation [N]" <- 0.0 ("AppliedForceTranslation")
      "AppliedForceRotation [N]" <- 0.0 ("AppliedForceRotation")
      "AbsolutePositionTranslation" <- 0.0
      "AbsolutePositionRotation" <- 0.0
      "AppliedTorqueRotation [Nmm]" <- 0.0 ("AppliedForceRotation")
      "SoftSafety" <- TRUE
      "HardSafety" <- TRUE
      "Case" <- 0
      "Save Data" <- FALSE
      "ForcePeak[N]" <- 0.0 ("ForcePeak[N]")
      "Reached" <- FALSE ("Reached")
      "Baseline[N]" <- 0.0 ("Baseline[N]")
      "NewPerturbation" <- TRUE ("NewPerturbation")
      "CalibratorTranslation" <- 0.0
      "CalibratorRotation" <- 0.0
      "Safety Been Triggered" <- FALSE
      "Safety Warning" <- FALSE
    }
    frame #1 {
      w50 = 62027
      w53 = 2.5
      w54 = 2.5
      w59 = 62025
      w62 = 62023
      w71 = 62021
      w74 = 62019
      w83 = 62017
      w86 = 62015
      w95 = 62013
      w98 = 62011
      # "Ensure motors command 2.5V at start-up (so motor current is 0A)"
      # "1: Initialzie UDP Connections"
      n12 = local read "IPAddress"() -> (w49:i64)
      n13 = local read "UDPTimestamp"() -> (w47:T1)
      n14 = local read "IPAddress"() -> (w61:i64)
      n15 = local read "UDPPerturbation"() -> (w56:T5)
      n16 = local read "IPAddress"() -> (w73:i64)
      n17 = local read "IPAddress"() -> (w72:i64)
      n18 = local read "UDPMotorData"() -> (w89:T5)
      n19 = local read "UDPConnection"() -> (w101:T5)
      n20 = local read "IPAddress"() -> (w97:i64)
      n21 = local read "UDPMode"() -> (w92:T5)
      n22 = local read "IPAddress"() -> (w96:i64)
      n23 = local read "IPAddress"() -> (w85:i64)
      n24 = local read "UDPCalibration"() -> (w80:T5)
      n25 = local read "IPAddress"() -> (w84:i64)
      n26 = local read "UDPMotorValues"() -> (w77:T5)
      n27 = local read "UDPSafety"() -> (w68:T5)
      n28 = local read "UDPGame"() -> (w65:T5)
      n29 = local read "IPAddress"() -> (w60:i64)
      n30 = UDP Open(11:w98) -> (port=w100:refnum<k16>)  [unwired: 4 in, 2 out]
      n31 = UDP Open(11:w86) -> (port=w88:refnum<k16>)  [unwired: 4 in, 2 out]
      n32 = UDP Open(11:w83) -> (port=w81:refnum<k16>)  [unwired: 4 in, 2 out]
      n33 = UDP Open(11:w74) -> (port=w76:refnum<k16>)  [unwired: 4 in, 2 out]
      n34 = UDP Open(11:w71) -> (port=w69:refnum<k16>)  [unwired: 4 in, 2 out]
      n35 = UDP Open(11:w62) -> (port=w64:refnum<k16>)  [unwired: 4 in, 2 out]
      n36 = UDP Open(11:w59) -> (port=w57:refnum<k16>)  [unwired: 4 in, 2 out]
      n37 = UDP Open(11:w50) -> (port=w52:refnum<k16>)  [unwired: 4 in, 2 out]
      n38 = UDP Open(11:w95) -> (port=w93:refnum<k16>)  [unwired: 4 in, 2 out]
      n39 = Bundle(cluster=w77, "UDP"=w76, "Receive Port"=w74, "Send Port"=62020, "Address"=w73) -> (→"UDPMotorValues":T5)
      n40 = Bundle(cluster=w101, "UDP"=w100, "Receive Port"=w98, "Send Port"=62012, "Address"=w97) -> (→"UDPConnection":T5)
      n41 = Bundle(cluster=w92, "UDP"=w93, "Receive Port"=w95, "Send Port"=62014, "Address"=w96) -> (→"UDPMode":T5)
      n42 = Bundle(cluster=w89, "UDP"=w88, "Receive Port"=w86, "Send Port"=62016, "Address"=w85) -> (→"UDPMotorData":T5)
      n43 = Bundle(cluster=w80, "UDP"=w81, "Receive Port"=w83, "Send Port"=62018, "Address"=w84) -> (→"UDPCalibration":T5)
      n44 = Bundle(cluster=w68, "UDP"=w69, "Receive Port"=w71, "Send Port"=62022, "Address"=w72) -> (→"UDPSafety":T5)
      n45 = Bundle(cluster=w56, "UDP"=w57, "Receive Port"=w59, "Send Port"=62026, "Address"=w60) -> (→"UDPPerturbation":T5)
      n46 = Bundle(cluster=w65, "UDP"=w64, "Receive Port"=w62, "Send Port"=62024, "Address"=w61) -> (→"UDPGame":T5)
      n47 = Bundle(cluster=w47, "port"=w52, w50, 62028, "IPAddress"=w49) -> (→"UDPTimestamp":T1)
      n48 = xnode "Analog output (1 sample)"("Motor1Current_AREAD (B/AO0 (Pin 2))"=w54, "Motor2Current_AREAD (A/AO0 (Pin 2))"=w53) -> ()  [unwired: 1 in, 1 out]
      "VoltageRotation" <- w53
      "VoltageTranslation" <- w54
    }
    frame #2 {
      # "Main brakes (24V) are open if set to TRUE\nSupport brakes resistors (brake switch) are open if set \nto TRUE and bring the main brake voltage to 16V, to\nsave energy and avoid overheat. Should be activated\nin the long term use.\n\nNote for RHK only: The BrakeSwitch 40 is left to FALSE  \nas it generates a voltage offset in the potentiometers\nwhen it is activated (TRUE)."
      # "2: Initialize Motors"
      n49 = call "Init Robot.vi"("Brake Switch 35"=FALSE, "Brake Switch 40"=FALSE, "Brake 40"=TRUE, "Brake 35"=TRUE) -> ("Force bias PS_R"=w144:dbl, "Force bias GR_R"=w145:dbl, "Force bias PS_L"=w146:dbl, "Force bias GR_L"=w150:dbl, "Right  Poti Initialise"=w158:dbl, "Left Poti Initialise"=w159:dbl, "Rot Poti Initialise"=w142:dbl)  [unwired: 1 in]
      "ForceBiasPS_L" <- w146
      "ForceBiasGR_L" <- w150
      "ForceBiasPS_R" <- w144
      "ForceBiasGR_R" <- w145
      n50 = local read "Right Poti Gradient"() -> (w155:dbl)
      n51 = local read "Right Poti Offset"() -> (w154:dbl)
      n52 = local read "Left Poti Gradient"() -> (w157:dbl)
      n53 = local read "Left Poti Offset"() -> (w156:dbl)
      n54 = call "Rot_pot_voltage_to_degree.vi"("RotaryPot (Voltage)"=w142) -> ("RotaryPot (degree)"=→"InitialRotation":dbl)
      n55 = call "Lin_pot_voltage_to_mm_Left.vi"("Offset"=w156, "Gradient"=w157, "LinPot Voltage"=w159) -> ("LinPot mm (center to finger)"=w149:dbl)  [unwired: 1 out]
      "LinPot mm (center to finger)" <- w149
      n56 = call "Lin_pot_voltage_to_mm_Right.vi"("Offset"=w154, "Gradient"=w155, "LinPot Voltage"=w158) -> ("LinPot mm (center to finger)"=w148:dbl)  [unwired: 1 out]
      "LinPot mm (center to finger) 2" <- w148
      n57 = Add(x=w149, y=w148) -> (x+y=w153:dbl)
      n58 = xnode "Digital output (1 sample) 4"("SIG_REL2 (B/DIO1 (Pin 13))"=TRUE, "SIG_REL4 (B/DIO3 (Pin 17))"=TRUE) -> ()  [unwired: 1 in, 1 out]
      n59 = Divide(x=w153, y=2.0) -> (x/y=→"InitialTranslation":dbl)
      n60 = call "InitialSensorCheck.vi"("LinPot mm (center to finger) RIGHT"=w148, "LinPot mm (center to finger) LEFT"=w149, "Force bias GR_L"=w150, "Force bias PS_R"=w144, "Force bias GR_R"=w145, "Force bias PS_L"=w146) -> ("Potentiometer Faulty"=→"Pots Faulty":bool, "Force Sensor Faulty"=→"Force Sensor Faulty":bool)  [unwired: 4 in]
      "define_dX_GR" <- TRUE ("define_dX_GR")
    }
    frame #3 {
      # "3: Main Loop"
      n61 = local read "Period"() -> (w208:i32)
      n62 = node-c288(w208) -> (w212:T26)  [unwired: 3 in]
      n63 = To Unsigned Byte Integer(number=u8 0) -> (unsigned 8bit integer=w204:u8)
      n64 = timed-loop {
        timing: w212 -> [_]
        timing-out: [_] -> w211
        shift-right: [w393] -> _
        shift-left: FALSE -> [w397]
        shift-right: [w399] -> _
        shift-left: FALSE -> [w394]
        shift-right: [w392] -> _
        shift-left: w204 -> [w398]
        shift-right: [w396] -> _
        shift-left: _ -> [w395]
        i -> [w400]
        stop <- _ stop-if-true
        n65 = node-c288() -> ()  [unwired: 1 in, 1 out]
        n66 = stacked-sequence {
          tunnel: w400 -> [_ w691]
          tunnel: [_ w678] -> w399
          tunnel: [_ w680] -> w393
          tunnel: w394 -> [_ w690]
          tunnel: [_ w689] -> w392
          tunnel: w398 -> [_ w688]
          tunnel: w397 -> [_ w686]
          tunnel: [_ w685] -> w396
          tunnel: w395 -> [_ w675]
          frame #0 {
            # "force to torque conversion"
            # "3.1: Read all Sensors"
            n67 = xnode "Analog input (1 sample)"() -> ("ForceSensor_READ1 (C/AI0 (AI0))"=w428:dbl, "ForceSensor_READ2 (C/AI1 (AI1))"=w429:dbl, "ForceSensor_READ3 (B/AI0 (Pin 3))"=w436:dbl, "ForceSensor_READ4 (B/AI1 (Pin 5))"=w435:dbl, "AI_lin_pot_left (A/AI0 (Pin 3))"=w447:dbl, "AI_lin_pot_right (A/AI1 (Pin 5))"=w446:dbl, "AI_rot_pot (A/AI2 (Pin 7))"=w445:dbl)  [unwired: 1 in, 1 out]
            n68 = xnode "Encoder"() -> ("Counter Value"=w462:i32)  [unwired: 2 in, 3 out]
            n69 = xnode "Encoder 2"() -> ("Counter Value"=w465:i32)  [unwired: 2 in, 3 out]
            n70 = Build Array(w447, w446, w445) -> (→"Potentiometers_array":dbl[])
            n71 = local read "InitialRotation"() -> (w455:dbl)
            n72 = local read "LoopTime"() -> (w484:dbl)
            n73 = local read "InitialTranslation"() -> (w458:dbl)
            n74 = local read "LoopTime"() -> (w483:dbl)
            n75 = local read "ForceBiasGR_L"() -> (w444:dbl)
            n76 = local read "ForceBiasGR_R"() -> (w453:dbl)
            n77 = local read "ForceBiasPS_R"() -> (w452:dbl)
            n78 = local read "ForceBiasPS_L"() -> (w443:dbl)
            n79 = Subtract(x=w436, y=w453) -> (x-y=w433:dbl)
            n80 = Subtract(x=w428, y=w444) -> (x-y=w434:dbl)
            n81 = local read "LX gradient"() -> (w404:dbl)
            n82 = local read "RX gradient"() -> (w403:dbl)
            n83 = Subtract(x=w435, y=w452) -> (x-y=w431:dbl)
            n84 = local read "RY gradient"() -> (w401:dbl)
            n85 = Subtract(x=w429, y=w443) -> (x-y=w432:dbl)
            n86 = local read "LY gradient"() -> (w402:dbl)
            n87 = Multiply(x=w434, y=w404) -> (x*y=w424:dbl)
            "Left F_x[N]" <- w424
            n88 = call "Encoder2Postition_Rotation.vi"("Signal from Encoder"=w465, "Initial Position"=w455) -> ("Postion Rot"=w456:dbl)  [unwired: 9 in]
            n89 = call "Encoder2Postition_Translation.vi"("Signal from Encoder"=w462, "Initial Position"=w458) -> ("Postion Trans"=w479:dbl)  [unwired: 9 in]
            n90 = Multiply(x=w433, y=w403) -> (x*y=w426:dbl)
            "Right F_x[N]" <- w426
            n91 = local read "CalibratorRotation"() -> (w478:dbl)
            n92 = local read "CalibratorTranslation"() -> (w477:dbl)
            n93 = Multiply(x=w431, y=w401) -> (x*y=w425:dbl)
            "Right F_y[N]" <- w425
            n94 = Multiply(x=2.0, y=w458) -> (x*y=w459:dbl)
            n95 = Multiply(x=w432, y=w402) -> (x*y=w423:dbl)
            "Left F_y[N]" <- w423
            n96 = Negate(x=w459) -> (-x=w461:dbl)
            n97 = Multiply(x=2.0, y=w479) -> (x*y=w451:dbl)
            n98 = Negate(x=w455) -> (-x=w457:dbl)
            n99 = Add(x=w461, y=w451) -> ()  [unwired: 1 out]
            n100 = Add(x=w457, y=w456) -> ()  [unwired: 1 out]
            n101 = call "Position_to_Velocity.vi"("Position"=w456, "d"=8.0354e-05, "LoopTime"=w484) -> ("Velocity"=w473:dbl)  [unwired: 7 in]
            n102 = call "Position_to_Velocity.vi"("Position"=w451, "d"=5.819e-06, "LoopTime"=w483) -> ("Velocity"=w474:dbl)  [unwired: 7 in]
            n103 = Add(x=w478, y=w456) -> (x+y=w454:dbl)
            n104 = Add(x=w477, y=w451) -> (x+y=w450:dbl)
            n105 = local read "AbsolutePositionRotation"() -> (w440:dbl)
            n106 = local write "RelativePositionRotation"(w454) -> ()
            n107 = local write "AbsolutePositionRotation"(w456) -> ()
            n108 = local write "VelocityRotation"(w473) -> ()
            n109 = local write "RelativePositionTranslation"(w450) -> ()
            n110 = local write "AbsolutePositionTranslation"(w451) -> ()
            n111 = local write "VelocityTranslation"(w474) -> ()
            n112 = call "Fx_Gravity_compensation.vi"("AbsolutePositionRotation"=w440, "Fx_to_filter"=w424) -> ("F_x[N] Gravity compensated"=w441:dbl)  [unwired: 8 in, 1 out]
            n113 = call "Fy_Gravity_compensation.vi"("AbsolutePositionRotation in"=w440, "Fy_to_filter"=w425) -> ("F_y[N] Gravity compensated 2"=w419:dbl)  [unwired: 8 in, 1 out]
            n114 = call "Fy_Gravity_compensation.vi"("AbsolutePositionRotation in"=w440, "Fy_to_filter"=w423) -> ("F_y[N] Gravity compensated 2"=w420:dbl)  [unwired: 8 in, 1 out]
            n115 = call "Fx_Gravity_compensation.vi"("AbsolutePositionRotation"=w440, "Fx_to_filter"=w426) -> ("F_x[N] Gravity compensated"=w442:dbl)  [unwired: 8 in, 1 out]
            n116 = local read "Pots Faulty"() -> (w407:bool)
            n117 = Bundle(cluster=T29 {"Position"=0.0, "Velocity"=0.0} ("PositionData Rotation"), "Position"=w456, "Velocity"=w473) -> (w472:T29)
            n118 = Bundle(cluster=T29 {"Position"=0.0, "Velocity"=0.0} ("PositionData Rotation"), "Position"=w451, "Velocity"=w474) -> (w471:T29)
            n119 = local read "AbsolutePositionTranslation"() -> (w470:dbl)
            n120 = Add(x=w420, y=w419) -> (x+y=w421:dbl)
            n121 = Add(x=w441, y=w442) -> (x+y=w438:dbl)
            n122 = local read "Potentiometers_array"() -> (w406:dbl[])
            n123 = local read "Force Sensor Faulty"() -> (w427:bool)
            n124 = Divide(x=w438, y=2.0) -> (x/y=w437:dbl)
            n125 = local read "Safety Been Triggered"() -> (w422:bool)
            n126 = call "Buffer.vi"("MaxSize"=50, "InputData"=w437) -> ("Buffer"=→"ForceTransBuffer[N]":ext[])  [unwired: 9 in]
            n127 = local read "AbsolutePositionRotation"() -> (w405:dbl)
            n128 = call "HardSafety.vi"("Safety Been Triggered"=w422, "Potentiometers"=w406, "Position From Rot Encoder"=w405, "Force Sensor Faulty"=w427, "Pots Diff Too Much At Init"=w407, "LY"=w423, "LX"=w424, "RY"=w425, "RX"=w426) -> ("HARD SAFETY"=w416:bool)  [unwired: 2 in]
            n129 = Not(x=w416) -> (.not. x?=w415:bool)
            n130 = local read "Mode"() -> (w418:T9)
            n131 = Divide(x=w470, y=2.0) -> (x/y=w468:dbl)
            n132 = local read "Mode"() -> (w411:T9)
            n133 = Equal?(x=w418, y=ModeControl."Run" ("Mode")) -> (x = y?=w412:bool)
            n134 = Equal?(x=w411, y=ModeControl."Safety" ("Mode")) -> (x = y?=w409:bool)
            n135 = Or(x=w412, y=w409) -> (x .or. y?=w408:bool)
            n136 = And(x=w415, y=w408) -> (x .and. y?=w414:bool)
            n137 = local write "AppliedForceTranslation [N]"(w438) -> ()
            n138 = local write "AppliedForceRotation [N]"(w421) -> ()
            n139 = Not(x=w414) -> (.not. x?=w413:bool)
            n140 = xnode "Digital output (1 sample) 5"("Motor1 dig 4 (B/DIO7 (Pin 25))"=TRUE, "Motor2 dig 4 (B/DIO9 (Pin 29))"=TRUE) -> ()  [unwired: 1 in, 1 out]
            n141 = case shown="False" w413 {
              frame False {
                n142 = local write "Safety Been Triggered"(TRUE) -> ()
                n143 = local write "Mode"(ModeControl."Safety" ("Mode")) -> ()
                n144 = local write "HardSafety"(FALSE) -> ()
              }
              frame True {
              }
            }
            n145 = Multiply(x=w421, y=w468) -> (x*y=w430:dbl)
            "Applied Torque Rotation" <- w430
            n146 = call "SoftSafety.vi"("PositionData Translation"=w471, "PositionData Rotation"=w472, "AppliedTorqueRotation"=w430, "AppliedForceTranslation"=w438) -> ("SoftSafety"=w449:bool)  [unwired: 3 in]
            n147 = case shown="True" w449 {
              frame True {
                n148 = local read "Safety Been Triggered"() -> (w660:bool)
                n149 = local read "Mode"() -> (w664:T9)
                n150 = Equal?(x=w664, y=ModeControl."Safety" ("Mode")) -> (x = y?=w661:bool)
                n151 = Not(x=w660) -> (.not. x?=w659:bool)
                n152 = Compound Arithmetic op=AND(w661, w659) -> (w662:bool)
                n153 = case shown="True" w662 {
                  frame False {
                  }
                  frame True {
                    n154 = local write "SoftSafety"(TRUE) -> ()
                    n155 = local write "Mode"(ModeControl."Run" ("Mode")) -> ()
                  }
                }
              }
              frame False {
                n156 = local read "Mode"() -> (w669:T9)
                n157 = Equal?(x=w669, y=ModeControl."Run" ("Mode")) -> (x = y?=w667:bool)
                n158 = case shown="True" w667 {
                  frame False {
                  }
                  frame True {
                    n159 = local write "SoftSafety"(FALSE) -> ()
                    n160 = local write "Mode"(ModeControl."Safety" ("Mode")) -> ()
                  }
                }
              }
            }
            n161 = local write "AppliedTorqueRotation [Nmm]"(w430) -> ()
          }
          frame #1 {
            # "3.2: Apply Brakes and Voltage"
            n162 = local read "Mode"() -> (w672:T9)
            n163 = case shown="\"Run\"" w672 {
              tunnel: [FALSE w781 TRUE ("manual brake grasping") TRUE FALSE] -> w678
              tunnel: [FALSE w780 TRUE ("Manual Break rotation") TRUE FALSE] -> w680
              tunnel: [2.5 ("output") 2.5 w799 2.5 ("output") 2.5 ("output")] -> w674
              tunnel: [2.5 ("output") w774 w798 2.5 ("output") 2.5 ("output")] -> w673
              tunnel: w691 -> [_ _ w803 _ _]
              frame "Wait", Default {
              }
              frame "Calibrate" {
                n164 = local read "Calibration"() -> (w784:T8)
                n165 = Unbundle(w784) -> ("CalibrationMode"=w783:enum16{"Wait", "Calibrate"}, "CalibratingMotor"=w782:i8)
                n166 = case shown="\"Calibrate\"" w783 {
                  tunnel: [FALSE w788] -> w780
                  tunnel: [FALSE w787] -> w781
                  tunnel: w782 -> [_ w789]
                  frame "Wait" {
                  }
                  frame "Calibrate" {
                    n167 = case shown="1" w789 {
                      tunnel: [TRUE FALSE] -> w788
                      tunnel: [FALSE TRUE] -> w787
                      frame 0, Default {
                      }
                      frame 1 {
                      }
                    }
                  }
                }
                n168 = local read "VelocityTranslation"() -> (w777:dbl)
                n169 = local read "AbsolutePositionTranslation"() -> (w778:dbl)
                n170 = call "SpringDamperForcePS.vi"("MotorVelocity"=w777, "MotorPosition"=w778, "SpringDampers"=T36 [{"startPosition"=47.0, "middlePosition"=42.0, "endPosition"=0.0, "forceConstant"=-140.0, "isDamper"=FALSE}, {"startPosition"=47.0, "middlePosition"=42.0, "endPosition"=0.0, "forceConstant"=3.0, "isDamper"=TRUE}]) -> ("Force"=w775:dbl)  [unwired: 1 in]
                n171 = call "Force2VoltageTrans.vi"("force"=w775) -> ("voltage"=w774:dbl)  [unwired: 10 in]
              }
              frame "Run" {
                w800 = 1 ("index")
                w808 = 0 ("index")
                n172 = local read "MotorData"() -> (w794:T7)
                n173 = local read "MotorData"() -> (w795:T7)
                n174 = Index Array(array=w794, index=w800) -> (element=w811:T38)
                n175 = Index Array(array=w795, index=w808) -> (element=w807:T38)
                n176 = Unbundle(w811) -> ("motorMode"=w796:enum16{"Stop", "Move", "Force", "Perturbation"}, "stopPosition"=w809:dbl, "velocityProfile"=w810:cluster{"position":dbl, "velocity":dbl}, "springDampers"=w812:T36, "Perturbation data"=w802:T42)
                n177 = Unbundle(w807) -> ("motorMode"=w797:enum16{"Stop", "Move", "Force", "Perturbation"}, "stopPosition"=w806:dbl, "velocityProfile"=w805:cluster{"position":dbl, "velocity":dbl}, "springDampers"=w804:T36, "Perturbation data"=w801:T42)
                n178 = case shown="\"Force\"" w796 {
                  tunnel: w809 -> [w816 _ _ _]
                  tunnel: [w819 w827 w887 w897] -> w798
                  tunnel: w810 -> [_ w829 _ _]
                  tunnel: w800 -> [_ w828 _ _]
                  tunnel: w812 -> [_ _ w892 _]
                  tunnel: w803 -> [_ _ _ w909]
                  tunnel: w802 -> [_ _ _ w904]
                  frame "Stop", Default {
                    # "Motor Voltage (0-5)V"
                    n179 = local write "define_dX_GR"(TRUE ("define_dX_GR")) -> ()
                    n180 = local write "Case"(0) -> ()
                    n181 = local read "RelativePositionTranslation"() -> (w818:dbl)
                    n182 = local read "LoopTime"() -> (w823:dbl)
                    n183 = call-poly <vilib>:"PID.vi"("output range"=cluster{"output high":dbl, "output low":dbl} {"output high"=2.5, "output low"=-2.5}, "dt (s)"=w823, "PID gains"=T37 {"proportional gain (Kc)"=2.5, "integral time (Ti, min)"=0.0, "derivative time (Td, min)"=0.0003}, "process variable"=w818, "setpoint"=w816) -> ("output"=w821:dbl)  [unwired: 5 in, 1 out]
                    n184 = Add(x=w821, y=2.5) -> (x+y=w819:dbl)
                  }
                  frame "Move" {
                    n185 = flat-sequence {
                      tunnel: w828 -> [w831]
                      tunnel: w829 -> [w832]
                      tunnel: [w832] -> w826
                      tunnel: [w831] -> w825
                      tunnel: [w840] -> w827
                      tunnel: w826 -> [w862]
                      tunnel: w825 -> [w861]
                      frame #0 {
                        n186 = local read "define_dX_GR"() -> (w830:bool)
                        n187 = case shown="True" w830 {
                          frame False {
                          }
                          frame True {
                            n188 = local read "RelativePositionTranslation"() -> (w833:dbl)
                            n189 = local write "dx GR (mm)"(w833) -> ()
                            n190 = local write "define_dX_GR"(FALSE ("define_dX_GR")) -> ()
                          }
                        }
                      }
                      frame #1 {
                        w854 = 0.01 ("y")
                        # "graph to compare setpoint and process variable in [mm]"
                        # "as long as \"dx GR\" is not equal to \ntarget position, \"dx GR\" is changed \neach frame depending on given velocity"
                        # "when target position is reached, change to \"stop mode\""
                        # "Motor Voltage"
                        # "relative velocity (desired)"
                        n191 = Unbundle(w862) -> ("position"=w846:dbl, "velocity"=w836:dbl)
                        n192 = local read "dx GR (mm)"() -> (w850:dbl)
                        n193 = Divide(x=1.0 ("y"), y=1000.0) -> (x/y=w852:dbl)
                        n194 = Add(x=w850, y=w854) -> (x+y=w855:dbl)
                        n195 = Subtract(x=w850, y=w854) -> (x-y=w856:dbl)
                        n196 = Multiply(x=w852, y=w836) -> (x*y=w843:dbl)
                        n197 = In Range and Coerce(upper limit=w855, x=w846, lower limit=w856) -> (In Range?=w849:bool)  [unwired: 1 out]
                        n198 = local read "RelativePositionTranslation"() -> (w847:dbl)
                        n199 = case shown="False" w849 {
                          tunnel: w850 -> [w866 w868]
                          tunnel: w843 -> [w865 _]
                          tunnel: [w867 w868] -> w845
                          frame False {
                            n200 = Add(x=w866, y=w865) -> (x+y=w867:dbl)
                          }
                          frame True {
                          }
                        }
                        n201 = local write "dx GR (mm)"(w845) -> ()
                        n202 = Bundle("RelativePositionTranslation"=w847, "dx GR (mm)"=w845) -> (→"GR Setpoint/ProcessVar [mm]":T43)  [unwired: 1 in]
                        n203 = Absolute Value(x=w836) -> (abs(x)=w837:dbl)
                        n204 = Greater?(x=w837, y=1.5) -> (0:w838:bool)
                        n205 = case shown="True" w838 {
                          tunnel: [T37 {"proportional gain (Kc)"=1.0, "integral time (Ti, min)"=0.0, "derivative time (Td, min)"=1e-06} ("PID gains mov slow") T37 {"proportional gain (Kc)"=2.5, "integral time (Ti, min)"=0.0, "derivative time (Td, min)"=0.0001} ("PID gains move fast")] -> w859
                          frame False {
                            # "\"low speed\" PID"
                          }
                          frame True {
                            # "normal speed PID"
                          }
                        }
                        n206 = local read "RelativePositionTranslation"() -> (w844:dbl)
                        n207 = local read "dx GR (mm)"() -> (w842:dbl)
                        n208 = case shown="True" w849 {
                          tunnel: w861 -> [_ w869]
                          tunnel: w846 -> [_ w871]
                          frame False {
                          }
                          frame True {
                            # "automatically change mode\nwhen target is reached"
                            n209 = local read "MotorData"() -> (w874:T7)
                            n210 = Index Array(array=w874, index=w869) -> (element=w875:T38)
                            n211 = Bundle(cluster=w875, "motorMode"=enum16{"Stop", "Move", "Force", "Perturbation"}."Stop" ("MotorMode"), "stopPosition"=w871) -> (w872:T38)  [unwired: 3 in]
                            n212 = Replace Array Subset(array=w874, new element=w872, index=w869) -> (w873:T7)
                            n213 = local write "MotorData"(w873) -> ()
                          }
                        }
                        n214 = local read "LoopTime"() -> (w860:dbl)
                        n215 = call-poly <vilib>:"PID.vi"("output range"=cluster{"output high":dbl, "output low":dbl} {"output high"=2.5, "output low"=-2.5}, "dt (s)"=w860, "PID gains"=w859, "process variable"=w844, "setpoint"=w842) -> ("output"=w839:dbl)  [unwired: 5 in, 1 out]
                        n216 = local write "Case"(0) -> ()
                        n217 = Add(x=w839, y=2.5) -> (x+y=w840:dbl)
                      }
                    }
                  }
                  frame "Force" {
                    w879 = 30.0 ("x")
                    w877 = 3.5 ("Kf_GR")
                    # "Giada: fade down kf from 3.5 at position 48\n until 0.2 at position 39 -> y = 0.3667 x-14.1\nPrima: y = 3/5x - 23.5"
                    # "Saturate force feedback to reduce instability"
                    # "Kf"
                    # "Force=sum of left and right horizontal forces, as for JC"
                    # "Velocity is 1/2 this in JC"
                    # "=1 in JC"
                    # "Kf=10 in JC"
                    n218 = local read "RelativePositionTranslation"() -> (w891:dbl)
                    n219 = local read "VelocityTranslation"() -> (w890:dbl)
                    n220 = call "SpringDamperForceGR.vi"("MotorVelocity"=w890, "MotorPosition"=w891, "SpringDampers"=w892) -> ("Force"=w876:dbl)  [unwired: 1 in]
                    n221 = local read "AppliedForceTranslation [N]"() -> (w881:dbl)
                    n222 = local write "define_dX_GR"(TRUE ("define_dX_GR")) -> ()
                    n223 = Negate(x=w879) -> (-x=w878:dbl)
                    n224 = In Range and Coerce(upper limit=w879, x=w881, lower limit=w878) -> (coerced(x)=w880:dbl)  [unwired: 1 out]
                    n225 = Add(x=1.0, y=w877) -> (x+y=w889:dbl)
                    n226 = Multiply(x=w877, y=w880) -> (x*y=w884:dbl)
                    n227 = Multiply(x=w876, y=w889) -> (x*y=w883:dbl)
                    n228 = Subtract(x=w883, y=w884) -> (x-y=w885:dbl)
                    n229 = call "Force2VoltageTrans.vi"("force"=w885) -> ("voltage"=w887:dbl)  [unwired: 10 in]
                    n230 = local write "Case"(0) -> ()
                  }
                  frame "Perturbation" {
                    # "Target Position"
                    n231 = local read "RelativePositionTranslation"() -> (w905:dbl)
                    n232 = Unbundle(w904) -> ("displacement"=w902:dbl, "timeInterval"=w901:dbl, "sign"=w903:i64)
                    n233 = local read "Case"() -> (w908:i32)
                    n234 = case shown="3" w908 {
                      tunnel: w909 -> [w922 w929 w951 w995 _]
                      tunnel: [w921 w926 w947 w992 w1003] -> w893
                      tunnel: w905 -> [w921 _ w948 w991 _]
                      tunnel: w903 -> [w914 w923 w945 w985 _]
                      tunnel: w902 -> [_ w925 _ w986 _]
                      tunnel: w901 -> [w913 w924 w944 _ _]
                      frame 0, Default {
                        # "Register time and position at beginning of perturbation ramp, and update baseline force value"
                        n235 = local read "ForceTransBuffer[N]"() -> (w919:ext[])
                        n236 = Add Array Elements(numeric array=w919) -> (sum=w917:ext)
                        n237 = local read "Perturbation"() -> (w916:T6)
                        n238 = Array Size(array=w919) -> (size(s)=w918:i32)
                        n239 = Divide(x=w917, y=w918) -> (x/y=w910:ext)
                        n240 = local write "Baseline[N]"(w910) -> ()
                        n241 = call "updatePerturbation.vi"("delta(T)/baseline(F)"=FALSE, "motor"=1, "timeInterval"=w913, "PertSign"=w914, "newValue"=w910, "perturbationIn"=w916) -> ("perturbationOut"=w915:T6)  [unwired: 5 in]
                        n242 = local write "Perturbation"(w915) -> ()
                        n243 = local write "Case"(1) -> ()
                        "isaved" <- w922
                        "Relative Pos Trans Saved" <- w921
                      }
                      frame 1 {
                        # "generate target ramp profile. Once reached, \nstore max force peak of last 50ms"
                        # "Sign"
                        # "Time Interval"
                        # "Displacement"
                        n244 = local read "isaved"() -> (w932:i32)
                        n245 = local read "Relative Pos Trans Saved"() -> (w927:dbl)
                        n246 = Multiply(x=w925, y=w923) -> (x*y=w928:dbl)
                        n247 = Subtract(x=w929, y=w932) -> (x-y=w931:i32)
                        n248 = Divide(x=w928, y=w924) -> (x/y=w934:dbl)
                        n249 = Greater?(x=w931, y=w924) -> (0:w930:bool)
                        n250 = Multiply(x=w934, y=w931) -> (x*y=w933:dbl)
                        n251 = Add(x=w927, y=w933) -> (x+y=w926:dbl)
                        n252 = case shown="True" w930 {
                          tunnel: w929 -> [_ w943]
                          tunnel: w926 -> [_ w941]
                          tunnel: w923 -> [_ w939]
                          frame False {
                          }
                          frame True {
                            n253 = local read "ForceTransBuffer[N]"() -> (w940:ext[])
                            n254 = local write "Relative Pos Trans Saved"(w941) -> ()
                            n255 = Greater Than 0?(x=w939) -> (x > 0?=w938:bool)
                            n256 = local write "isaved"(w943) -> ()
                            n257 = Array Max & Min(array=w940) -> (max value=w937:ext, min value=w936:ext)  [unwired: 2 out]
                            n258 = Select(t=w937, s=w938, f=w936) -> (s? t:f=w935:ext)
                            n259 = local write "ForcePeak[N]"(w935) -> ()
                            n260 = local write "Case"(2) -> ()
                          }
                        }
                      }
                      frame 2 {
                        # "hold top of ramp for 100ms"
                        n261 = local read "isaved"() -> (w952:i32)
                        n262 = Subtract(x=w951, y=w952) -> (x-y=w946:i32)
                        n263 = local read "Relative Pos Trans Saved"() -> (w947:dbl)
                        n264 = Greater?(x=w946, y=100) -> (0:w949:bool)
                        n265 = case shown="True" w949 {
                          tunnel: w951 -> [_ w983]
                          tunnel: w948 -> [_ w982]
                          tunnel: w946 -> [w959 _]
                          tunnel: w945 -> [w953 w974]
                          tunnel: w944 -> [_ w973]
                          frame False {
                            # "50ms after the top of the ramp, evaluate the\nforce peak (-50ms before to +50ms after the ramp top)"
                            n266 = local read "Reached"() -> (w955:bool)
                            n267 = Greater?(x=w959, y=50.0) -> (0:w957:bool)
                            n268 = Not(x=w955) -> (.not. x?=w956:bool)
                            n269 = And(x=w957, y=w956) -> (x .and. y?=w954:bool)
                            n270 = case shown="True" w954 {
                              tunnel: w953 -> [_ w966]
                              frame False {
                              }
                              frame True {
                                # "verify if the force peak was before the ramp end\n(ForcePeak) or after (from last ForceTransBuffer)"
                                n271 = local read "ForceTransBuffer[N]"() -> (w967:ext[])
                                n272 = Greater Than 0?(x=w966) -> (x > 0?=w963:bool)
                                n273 = local read "ForcePeak[N]"() -> (w964:dbl)
                                n274 = Array Max & Min(array=w967) -> (max value=w969:ext, min value=w968:ext)  [unwired: 2 out]
                                n275 = Select(t=w969, s=w963, f=w968) -> (s? t:f=w965:ext)
                                n276 = Max & Min(x=w965, y=w964) -> (max(x,y)=w962:ext, min(x,y)=w961:ext)
                                n277 = Select(t=w962, s=w963, f=w961) -> (s? t:f=w960:ext)
                                n278 = local write "ForcePeak[N]"(w960) -> ()
                                n279 = local write "Reached"(TRUE ("Reached")) -> ()
                              }
                            }
                          }
                          frame True {
                            # "switch to return phase (3, from top of ramp to baseline position)\nand save the perturbation-induced delta force in Perturbation data"
                            n280 = local read "ForcePeak[N]"() -> (w980:dbl)
                            n281 = local read "Baseline[N]"() -> (w979:dbl)
                            n282 = local write "isaved"(w983) -> ()
                            n283 = Subtract(x=w980, y=w979) -> (x-y=w978:dbl)
                            n284 = local read "Perturbation"() -> (w977:T6)
                            n285 = local write "Relative Pos Trans Saved"(w982) -> ()
                            n286 = call "updatePerturbation.vi"("delta(T)/baseline(F)"=TRUE, "motor"=1, "timeInterval"=w973, "PertSign"=w974, "newValue"=w978, "perturbationIn"=w977) -> ("perturbationOut"=w976:T6)  [unwired: 5 in]
                            n287 = local write "Perturbation"(w976) -> ()
                            n288 = local write "Reached"(FALSE ("Reached")) -> ()
                            n289 = local write "NewPerturbation"(TRUE ("NewPerturbation")) -> ()
                            n290 = local write "Case"(3) -> ()
                          }
                        }
                      }
                      frame 3 {
                        # "return to start position in 900ms"
                        # "Sign"
                        # "Displacement"
                        n291 = local read "Relative Pos Trans Saved"() -> (w987:dbl)
                        n292 = local read "isaved"() -> (w997:i32)
                        n293 = Multiply(x=w986, y=w985) -> (x*y=w990:dbl)
                        n294 = Divide(x=w990, y=900.0) -> (x/y=w996:dbl)
                        n295 = Subtract(x=w995, y=w997) -> (x-y=w989:i32)
                        n296 = Multiply(x=w996, y=w989) -> (x*y=w988:dbl)
                        n297 = Greater?(x=w989, y=900) -> (0:w993:bool)
                        n298 = Subtract(x=w987, y=w988) -> (x-y=w992:dbl)
                        n299 = case shown="True" w993 {
                          tunnel: w995 -> [_ w1001]
                          tunnel: w991 -> [_ w999]
                          frame False {
                          }
                          frame True {
                            n300 = local write "Relative Pos Trans Saved"(w999) -> ()
                            n301 = local write "Case"(4) -> ()
                            n302 = local write "isaved"(w1001) -> ()
                          }
                        }
                      }
                      frame 4 {
                        w1002 = 1
                        # "command return to stop mode"
                        n303 = local read "RelativePositionTranslation"() -> (w1003:dbl)
                        n304 = local read "MotorData"() -> (w1008:T7)
                        n305 = Index Array(array=w1008, index=w1002) -> (element=w1006:T38)
                        n306 = Bundle(cluster=w1006, "motorMode"=enum16{"Stop", "Move", "Force", "Perturbation"}."Stop" ("MotorMode"), "stopPosition"=w1003) -> (w1004:T38)  [unwired: 3 in]
                        n307 = Replace Array Subset(array=w1008, new element=w1004, index=w1002) -> (w1007:T7)
                        n308 = local write "MotorData"(w1007) -> ()
                      }
                    }
                    "Target Position Translation" <- w893
                    n309 = local write "define_dX_GR"(TRUE ("define_dX_GR")) -> ()
                    n310 = local read "LoopTime"() -> (w907:dbl)
                    n311 = local read "RelativePositionTranslation"() -> (w894:dbl)
                    n312 = Bundle("RelativePositionTranslation"=w894, "RelativePositionTranslation"=w893) -> (w895:T44)  [unwired: 1 in]
                    n313 = local write "GR Setpoint/ProcessVar [mm]"(w895) -> ()
                    n314 = call-poly <vilib>:"PID.vi"("output range"=cluster{"output high":dbl, "output low":dbl} {"output high"=2.5, "output low"=-2.5}, "dt (s)"=w907, "PID gains"=T37 {"proportional gain (Kc)"=2.5, "integral time (Ti, min)"=0.0, "derivative time (Td, min)"=0.0003}, "process variable"=w894, "setpoint"=w893) -> ("output"=w896:dbl)  [unwired: 5 in, 1 out]
                    n315 = Add(x=w896, y=2.5) -> (x+y=w897:dbl)
                  }
                }
                n316 = case shown="\"Force\"" w797 {
                  tunnel: w806 -> [w1009 _ _ _]
                  tunnel: [w1014 w1036 w1068 0.0] -> w799
                  tunnel: w805 -> [_ w1042 _ _]
                  tunnel: w808 -> [_ w1041 _ _]
                  tunnel: w804 -> [_ _ w1071 _]
                  tunnel: w801 -> [_ _ _ _]
                  frame "Stop", Default {
                    (unwired) T37 {"proportional gain (Kc)"=2.0, "integral time (Ti, min)"=0.0, "derivative time (Td, min)"=0.0005} ("PID gains")
                    # "RHK old gains"
                    n317 = local read "RelativePositionRotation"() -> (w1010:dbl)
                    n318 = local read "LoopTime"() -> (w1016:dbl)
                    n319 = call-poly <vilib>:"PID.vi"("output range"=cluster{"output high":dbl, "output low":dbl} {"output high"=2.5, "output low"=-2.5}, "dt (s)"=w1016, "PID gains"=T37 {"proportional gain (Kc)"=0.15, "integral time (Ti, min)"=0.0, "derivative time (Td, min)"=0.0004}, "process variable"=w1010, "setpoint"=w1009) -> ("output"=w1013:dbl)  [unwired: 5 in, 1 out]
                    n320 = Negate(x=w1013) -> (-x=w1012:dbl)
                    n321 = Add(x=w1012, y=2.5) -> (x+y=w1014:dbl)
                    "dtheta PS (deg)" <- w1009
                  }
                  frame "Move" {
                    w1029 = 0.01 ("y")
                    # "graph to compare setpoint and process variable in [mm]"
                    # "relative velocity (desired)"
                    # "as long as \"dtheta PS\" is not equal to \ntarget position, \"dtheta PS\" is changed \neach frame depending on given velocity"
                    # "when target position is reached, change to \"stop mode\""
                    n322 = Unbundle(w1042) -> ("position"=w1021:dbl, "velocity"=w1022:dbl)
                    n323 = local read "dtheta PS (deg)"() -> (w1025:dbl)
                    n324 = Divide(x=1.0 ("y"), y=1000.0) -> (x/y=w1027:dbl)
                    n325 = Add(x=w1025, y=w1029) -> (x+y=w1030:dbl)
                    n326 = Subtract(x=w1025, y=w1029) -> (x-y=w1031:dbl)
                    n327 = Multiply(x=w1027, y=w1022) -> (x*y=w1024:dbl)
                    n328 = In Range and Coerce(upper limit=w1030, x=w1021, lower limit=w1031) -> (In Range?=w1023:bool)  [unwired: 1 out]
                    n329 = case shown="False" w1023 {
                      tunnel: w1025 -> [w1044 w1046]
                      tunnel: w1024 -> [w1043 _]
                      tunnel: [w1045 w1046] -> w1019
                      frame False {
                        n330 = Add(x=w1044, y=w1043) -> (x+y=w1045:dbl)
                      }
                      frame True {
                      }
                    }
                    n331 = local write "dtheta PS (deg)"(w1019) -> ()
                    n332 = local read "RelativePositionRotation"() -> (w1018:dbl)
                    n333 = case shown="True" w1023 {
                      tunnel: w1041 -> [_ w1047]
                      tunnel: w1021 -> [_ w1049]
                      frame False {
                      }
                      frame True {
                        # "automatically change mode\nwhen target is reached"
                        n334 = local read "MotorData"() -> (w1052:T7)
                        n335 = Index Array(array=w1052, index=w1047) -> (element=w1053:T38)
                        n336 = Bundle(cluster=w1053, "motorMode"=enum16{"Stop", "Move", "Force"}."Stop" ("MotorMode"), "stopPosition"=w1049) -> (w1050:T38)  [unwired: 3 in]
                        n337 = Replace Array Subset(array=w1052, new element=w1050, index=w1047) -> (w1051:T7)
                        n338 = local write "MotorData"(w1051) -> ()
                      }
                    }
                    n339 = Bundle("RelativePositionRotation"=w1018, "dtheta PS (deg)"=w1019) -> (→"PS Setpoint/ProcessVar [mm]":T45)  [unwired: 1 in]
                    n340 = local read "RelativePositionRotation"() -> (w1040:dbl)
                    n341 = local read "dtheta PS (deg)"() -> (w1035:dbl)
                    n342 = local read "LoopTime"() -> (w1039:dbl)
                    n343 = call-poly <vilib>:"PID.vi"("output range"=cluster{"output high":dbl, "output low":dbl} {"output high"=2.5, "output low"=-2.5}, "dt (s)"=w1039, "PID gains"=T37 {"proportional gain (Kc)"=0.15, "integral time (Ti, min)"=0.0, "derivative time (Td, min)"=0.0004}, "process variable"=w1040, "setpoint"=w1035) -> ("output"=w1033:dbl)  [unwired: 5 in, 1 out]
                    n344 = Negate(x=w1033) -> (-x=w1032:dbl)
                    n345 = Add(x=w1032, y=2.5) -> (x+y=w1036:dbl)
                  }
                  frame "Force" {
                    # "rigid contact at 100deg and -100deg (spring + dumper)"
                    # "Resultant Torque desired in Nmm"
                    n346 = local read "AbsolutePositionRotation"() -> (w1067:dbl)
                    n347 = local read "VelocityRotation"() -> (w1066:dbl)
                    n348 = call "SpringDamperForcePS.vi"("MotorVelocity"=w1066, "MotorPosition"=w1067, "SpringDampers"=T36 [{"startPosition"=100.0, "middlePosition"=110.0, "endPosition"=300.0, "forceConstant"=-2000.0, "isDamper"=FALSE}, {"startPosition"=100.0, "middlePosition"=110.0, "endPosition"=300.0, "forceConstant"=10.0, "isDamper"=TRUE}, {"startPosition"=-100.0, "middlePosition"=-110.0, "endPosition"=-300.0, "forceConstant"=-2000.0, "isDamper"=FALSE}, {"startPosition"=-100.0, "middlePosition"=-110.0, "endPosition"=-300.0, "forceConstant"=10.0, "isDamper"=TRUE}] ("springDampers")) -> ("Force"=w1058:dbl)  [unwired: 1 in]
                    n349 = local read "RelativePositionRotation"() -> (w1070:dbl)
                    n350 = local read "VelocityRotation"() -> (w1069:dbl)
                    n351 = local read "AppliedTorqueRotation [Nmm]"() -> (w1061:dbl)
                    n352 = call "SpringDamperForcePS.vi"("MotorVelocity"=w1069, "MotorPosition"=w1070, "SpringDampers"=w1071) -> ("Force"=w1055:dbl)  [unwired: 1 in]
                    n353 = Add(x=w1055, y=w1058) -> (x+y=w1063:dbl)
                    n354 = Multiply(x=w1061, y=2.0) -> (x*y=w1056:dbl)
                    n355 = Negate(x=w1056) -> (-x=w1057:dbl)
                    n356 = Multiply(x=w1063, y=2.0) -> (x*y=w1064:dbl)
                    n357 = Subtract(x=w1064, y=w1057) -> (x-y=w1059:dbl)
                    n358 = Negate(x=w1059) -> (-x=w1060:dbl)
                    n359 = call "Torque2VoltageRot.vi"("torque"=w1060) -> ("voltage"=w1068:dbl)  [unwired: 10 in]
                  }
                  frame "Perturbation" {
                    # "Perturbation not implemented in pronosupination"
                    "Target Position Rotation" <- 0.0
                  }
                }
              }
              frame "Safety" {
              }
              frame "Quit" {
                # "when the Quit button of the patient selection (main window) is pressed to close\nUnity, go to Quit mode, which stops labview too"
                n360 = local write "Finalize"(TRUE ("Finalize")) -> ()
              }
            }
            "PID output voltage rotation" <- w674
            "PID output voltage translation" <- w673
            n361 = local read "Main Loop Time"() -> (w687:i32)
            n362 = local read "Main Loop Time"() -> (w684:i32)
            n363 = In Range and Coerce(upper limit=5.0, x=w674, lower limit=0.0) -> (coerced(x)=w676:dbl)  [unwired: 1 out]
            n364 = In Range and Coerce(upper limit=5.0, x=w673, lower limit=0.0) -> (coerced(x)=w677:dbl)  [unwired: 1 out]
            n365 = call "BrakeSwitchCommander.vi"("CurrentTick"=w687, "TickMemoryIn"=w688, "BrakeStateOld"=w690, "BrakeStateNew"=w678) -> ("TickMemoryOut"=w689:dbl, "BrakeSwitch Control"=w679:bool)  [unwired: 6 in]
            n366 = call "BrakeSwitchCommander.vi"("CurrentTick"=w684, "TickMemoryIn"=w675, "BrakeStateOld"=w686, "BrakeStateNew"=w680) -> ("TickMemoryOut"=w685:dbl, "BrakeSwitch Control"=w681:bool)  [unwired: 6 in]
            n367 = local write "VoltageTranslation"(w677) -> ()
            n368 = local write "VoltageRotation"(w676) -> ()
            n369 = xnode "Analog output (1 sample)"("MotorCtrl2 (A/AO0 (Pin 2))"=w677, "MotorCtrl1 (B/AO0 (Pin 2))"=w676) -> ()  [unwired: 1 in, 1 out]
            n370 = xnode "Digital output (1 sample)"("SIG_REL2 (B/DIO1 (Pin 13))"=w681, "SIG_REL3 (B/DIO2 (Pin 15))"=w680, "SIG_REL4 (B/DIO3 (Pin 17))"=w679, "SIG_REL5 (B/DIO4 (Pin 19))"=w678) -> ()  [unwired: 1 in, 1 out]
          }
        }
        n371 = local read "HardSafety"() -> (w391:bool)
        n372 = Not(x=w391) -> ()  [unwired: 1 out]
        n373 = node-c288() -> ()  [unwired: 1 in, 1 out]
        "Main Loop Time" <- w400
      }
      n374 = node-c288() -> (w210:T26)  [unwired: 4 in]
      n375 = node-c288() -> (w214:T26)  [unwired: 4 in]
      n376 = timed-loop {
        timing: w210 -> [_]
        timing-out: [_] -> w209
        shift-right: [w229] -> _
        shift-left: TypeDef_TDMS_States."Do Nothing" ("TDMS States") -> [w228]
        shift-right: [w227] -> _
        shift-left: _ -> [w226]
        shift-right: [w225] -> _
        shift-left: _ -> [w224]
        stop <- w215 stop-if-true
        # "Note: save data if either \nmanual SaveData or Game\nsaving are enabled. \nStop saving and close data file if\nboth Game saving and manual\nsaving are disabled, or if finalize\nbecomes true (=quit GUI or\nhard safety)"
        n377 = node-c288() -> ()  [unwired: 1 in, 1 out]
        n378 = local read "Game"() -> (w222:T4)
        n379 = local read "Finalize"() -> (w219:bool)
        n380 = Unbundle(w222) -> ("gameMode"=w221:T3)  [unwired: 4 out]
        n381 = Not(x=w219) -> (.not. x?=w218:bool)
        n382 = Not Equal To 0?(x=w221) -> (x != 0?=w220:bool)
        n383 = Or(x="SaveData (Manual)", y=w220) -> (x .or. y?=w217:bool)
        n384 = And(x=w217, y=w218) -> (x .and. y?=w216:bool)
        n385 = case shown="\"Create\"" w228 {
          selector: w228 -> [w234 _ _ _]
          tunnel: w216 -> [w236 w240 w274 _]
          tunnel: [w235 w242 w272 w381] -> w229
          tunnel: [w232 w243 w271 _] -> w227
          tunnel: w226 -> [w232 _ w275 w380]
          tunnel: [w231 w241 w270 w378] -> w225
          tunnel: w224 -> [w231 _ _ w379]
          tunnel: [w230 FALSE ("Finalize") FALSE ("Finalize") w376] -> w215
          frame "Do Nothing" {
            n386 = Select(t=TypeDef_TDMS_States."Create" ("TDMS States"), s=w236, f=w234) -> (s? t:f=w235:T24)
            n387 = local write "Save Data"(FALSE ("Save Data")) -> ()
            n388 = local read "Finalize"() -> (w230:bool)
          }
          frame "Create" {
            # "first you need to close the\nopen tdms file you started,\nthen you can quit labview"
            n389 = flat-sequence {
              tunnel: [w248] -> w241
              tunnel: [w247] -> w243
              tunnel: [w266] -> w242
              tunnel: w240 -> [w264]
              frame #0 {
                # "Create file \"ExerciseData_<Date Time>.tdms\""
                n390 = local read "TimeStampData"() -> (w244:cluster{"time":string})
                n391 = call <vilib>:"Check if File or Folder Exists.vi"("path"=path "U:/") -> ("error out"=w255:errorcluster, "file or folder exists?"=w257:bool, "dup path"=w256:path)  [unwired: 8 in]
                n392 = case shown="True" w257 {
                  tunnel: w256 -> [w261 w262]
                  tunnel: [w260 w263] -> w249
                  tunnel: w255 -> [w259 w263]
                  tunnel: [w258 w262] -> w245
                  frame False {
                    n393 = Create Folder(path (use dialog)=w261, error in=w259) -> (created path=w258:path, error out=w260:errorcluster)  [unwired: 1 in, 1 out]
                  }
                  frame True {
                  }
                }
                n394 = call "NameFileFromTimestamp.vi"("TimeStampData"=w244) -> ("String"=w254:string)  [unwired: 10 in]
                n395 = Build Path(base path=w245, name or relative path=w254) -> (appended path=w253:path)
                n396 = TDMS Open(5:TRUE, 7:enum16{"1.0", "2.0"}."2.0" ("file format version (2.0)"), 8:w249, 10:T25."create or replace" ("operation (0:open)"), 11:w253) -> (0:w248:errorcluster, 3:w247:refnum<k34>)  [unwired: 2 in]
              }
              frame #1 {
                n397 = Not(x=w264) -> (.not. x?=w265:bool)
                n398 = Select(t=TypeDef_TDMS_States."Close" ("TDMS States"), s=w265, f=TypeDef_TDMS_States."Write" ("TDMS States")) -> (s? t:f=w266:T24)
              }
            }
            n399 = local write "Save Data"(FALSE ("Save Data")) -> ()
          }
          frame "Write" {
            # "first you need to close the\nopen tdms file you started,\nthen you can quit labview"
            n400 = flat-sequence {
              tunnel: w275 -> [w357]
              tunnel: w274 -> [w356]
              tunnel: [w356] -> w273
              tunnel: [w338] -> w271
              tunnel: [w337] -> w270
              tunnel: w273 -> [w372]
              tunnel: [w371] -> w272
              frame #0 {
                n401 = local read "Right F_y[N]"() -> (w282:dbl)
                n402 = local read "Right F_x[N]"() -> (w283:dbl)
                n403 = local read "Left F_y[N]"() -> (w284:dbl)
                n404 = local read "Left F_x[N]"() -> (w285:dbl)
                n405 = local read "MotorData"() -> (w370:T7)
                n406 = local read "Perturbation"() -> (w332:T6)
                n407 = local read "Target Position Rotation"() -> (w333:dbl)
                n408 = local read "Main Loop Time"() -> (w363:i32)
                n409 = local read "RelativePositionTranslation"() -> (w280:dbl)
                n410 = local read "AbsolutePositionTranslation"() -> (w279:dbl)
                n411 = local read "MotorData"() -> (w366:T7)
                n412 = local read "AbsolutePositionRotation"() -> (w277:dbl)
                n413 = local read "RelativePositionRotation"() -> (w278:dbl)
                n414 = local read "Perturbation"() -> (w300:T6)
                n415 = local read "Target Position Translation"() -> (w311:dbl)
                n416 = Index Array(array=w366, index=1) -> (element=w364:T38)
                n417 = Index Array(array=w370, index=0) -> (element=w368:T38)
                n418 = Index Array(array=w332, index=0) -> (element=w330:T39)
                n419 = Unbundle(w364) -> ("motorMode"=w360:enum16{"Stop", "Move", "Force", "Perturbation"}, "stopPosition"=w343:dbl, "velocityProfile"=w352:cluster{"position":dbl, "velocity":dbl}, "springDampers"=w351:T36, "Perturbation data"=w359:T42)
                n420 = Index Array(array=w300, index=1) -> (element=w298:T39)
                n421 = Unbundle(w368) -> ("motorMode"=w367:enum16{"Stop", "Move", "Force", "Perturbation"}, "stopPosition"=w320:dbl, "velocityProfile"=w354:cluster{"position":dbl, "velocity":dbl}, "springDampers"=w353:T36, "Perturbation data"=w362:T42)
                n422 = Build Array(w285, w284, w283, w282) -> (w281:dbl[])
                n423 = Build Array(w280, w279, w278, w277) -> (w276:dbl[])
                n424 = Unbundle(w362) -> ("displacement"=w347:dbl, "timeInterval"=w346:dbl, "sign"=w361:i64)
                n425 = Unbundle(w359) -> ("displacement"=w350:dbl, "timeInterval"=w349:dbl, "sign"=w358:i64)
                n426 = Unbundle(w298) -> ("deltaOS"=w297:dbl, "baselineOS"=w296:dbl, "deltaOF"=w295:dbl, "baselineOF"=w294:dbl, "deltaCS"=w293:dbl, "baselineCS"=w292:dbl, "deltaCF"=w291:dbl, "baselineCF"=w290:dbl)
                n427 = To Double Precision Float(number=w363) -> (double precision float=w336:dbl)
                n428 = Unbundle(w330) -> ("deltaOS"=w329:dbl, "baselineOS"=w328:dbl, "deltaOF"=w327:dbl, "baselineOF"=w326:dbl, "deltaCS"=w325:dbl, "baselineCS"=w324:dbl, "deltaCF"=w323:dbl, "baselineCF"=w322:dbl)
                n429 = Unbundle(w354) -> ("position"=w319:dbl, "velocity"=w318:dbl)
                n430 = Unbundle(w352) -> ("position"=w342:dbl, "velocity"=w341:dbl)
                n431 = To Double Precision Float(number=w367) -> (double precision float=w321:dbl)
                n432 = To Double Precision Float(number=w358) -> (double precision float=w348:dbl)
                n433 = To Double Precision Float(number=w361) -> (double precision float=w345:dbl)
                n434 = To Double Precision Float(number=w360) -> (double precision float=w344:dbl)
                n435 = Build Array(w329, w328, w327, w326, w325, w324, w323, w322) -> (w314:dbl[])
                n436 = Build Array(w297, w296, w295, w294, w293, w292, w291, w290) -> (w289:dbl[])
                n437 = call "ExtractSpringDampers.vi"("SpringDampers"=w353) -> ("SpringDampersDataOut"=w316:dbl[])  [unwired: 4 in]
                n438 = Build Array(w347, w346, w345, w333) -> (w315:dbl[])
                n439 = Build Array(w321, w320, w319, w318) -> (w317:dbl[])
                n440 = call "ExtractSpringDampers.vi"("SpringDampers"=w351) -> ("SpringDampersDataOut"=w312:dbl[])  [unwired: 4 in]
                n441 = Build Array(w344, w343, w342, w341) -> (w313:dbl[])
                n442 = Build Array(w350, w349, w348, w311) -> (w310:dbl[])
                n443 = local read "HardSafety"() -> (w335:bool)
                n444 = local read "SoftSafety"() -> (w304:bool)
                n445 = local read "Mode"() -> (w286:T9)
                n446 = local read "Game"() -> (w340:T4)
                n447 = local read "Potentiometers_array"() -> (w301:dbl[])
                n448 = local write "Save Data"(TRUE ("Save Data")) -> ()
                n449 = Unbundle(w340) -> ("gameMode"=w339:T3, "level"=w308:dbl, "correctAnswers"=w307:dbl, "totalAnswers"=w306:dbl, "repetitions"=w305:dbl)
                n450 = Boolean To (0,1)(Boolean=w335) -> (0, 1=w302:i16)
                n451 = Boolean To (0,1)(Boolean=w304) -> (0, 1=w303:i16)
                n452 = To Double Precision Float(number=w339) -> (double precision float=w309:dbl)
                n453 = Build Array(w286, w309, w308, w307, w306, w305) -> (w288:dbl[])
                n454 = Build Array (concatenate)(w303, w302, w301) -> (w287:dbl[])
                n455 = Build Array (concatenate)(w336, w281, w276, w317, w316, w315, w314, w313, w312, w310, w289, w288, w287) -> (w334:dbl[])
                n456 = call "Save_Data_In_TDMS.vi"("tdms file"=w357, "Save Data"=w356, "data"=w334) -> ("error out"=w337:errorcluster, "tdms file out"=w338:refnum<k34>)  [unwired: 7 in]
              }
              frame #1 {
                n457 = Not(x=w372) -> (.not. x?=w373:bool)
                n458 = Select(t=TypeDef_TDMS_States."Close" ("TDMS States"), s=w373, f=TypeDef_TDMS_States."Write" ("TDMS States")) -> (s? t:f=w371:T24)
              }
            }
          }
          frame "Close" {
            n459 = flat-sequence {
              tunnel: w380 -> [w384]
              tunnel: [w383] -> w378
              tunnel: w379 -> [w382]
              tunnel: [TypeDef_TDMS_States."Do Nothing" ("TDMS States")] -> w381
              tunnel: [w385] -> w376
              frame #0 {
                n460 = TDMS Close(8:w382, 11:w384) -> (0:w383:errorcluster)  [unwired: 1 out]
              }
              frame #1 {
                # "After closing the last tdsm file, if Finalize is selected (quit \nGUI or hard safety), stop saving loop and quit labview.\nNote: Finalize stops loop in the \"do nothing\" or \"closing\", so any\nlast tdms file must be correctly saved before stopping labview"
                n461 = local read "Finalize"() -> (w385:bool)
              }
            }
            n462 = local write "Save Data"(FALSE ("Save Data")) -> ()
          }
        }
        n463 = node-c288() -> ()  [unwired: 1 in, 1 out]
      }
      n464 = timed-loop {
        timing: w214 -> [_]
        timing-out: [_] -> w213
        stop <- _ stop-if-true
        n465 = node-c288() -> ()  [unwired: 1 in, 1 out]
        n466 = stacked-sequence {
          frame #0 {
            # "Connection Check"
            n467 = local read "UDPConnection"() -> (w1091:T5)
            n468 = call "ReceiveFloat.vi"("UDP Input"=w1091) -> ("Did Receive"=w1089:bool, "UDP Output"=w1090:T5)  [unwired: 3 in, 2 out]
            n469 = local write "UDPConnection"(w1090) -> ()
            n470 = case shown="True" w1089 {
              frame False {
              }
              frame True {
                n471 = local read "UDPConnection"() -> (w1094:T5)
                n472 = local read "Mode"() -> (w1092:T9)
                n473 = To Double Precision Float(number=w1092) -> (double precision float=w1093:dbl)
                n474 = call "SendFloat.vi"("Sent Data"=w1093, "UDP Input"=w1094) -> ("UDP Output"=w1095:T5)  [unwired: 4 in, 1 out]
                n475 = local write "UDPConnection"(w1095) -> ()
              }
            }
          }
          frame #1 {
            # "Change Mode"
            n476 = local read "UDPMode"() -> (w1100:T5)
            n477 = call "ReceiveFloat.vi"("UDP Input"=w1100) -> ("Received Data"=w1098:dbl, "Did Receive"=w1096:bool, "UDP Output"=w1099:T5)  [unwired: 3 in, 1 out]
            n478 = To Word Integer(number=w1098) -> (16bit integer=w1102:i16)
            n479 = Type Cast(type=ModeControl."Wait" ("Mode"), x=w1102) -> (*(type *) &x=w1101:T9)
            n480 = local write "UDPMode"(w1099) -> ()
            n481 = case shown="True" w1096 {
              tunnel: w1101 -> [_ w1107]
              frame False {
              }
              frame True {
                n482 = case shown="\"Run\"" w1107 {
                  selector: w1107 -> [w1108 w1113 w1123 _ w1127]
                  tunnel: [w1108 w1113 w1123 w1126 w1127] -> w1103
                  frame "Wait", Default {
                  }
                  frame "Calibrate" {
                    n483 = local read "Calibration"() -> (w1112:T8)
                    n484 = Bundle(cluster=w1112, "CalibrationMode"=enum16{"Wait", "Calibrate"}."Wait", "CalibratingMotor"=i8 0) -> (w1111:T8)
                    n485 = local write "Calibration"(w1111) -> ()
                  }
                  frame "Run" {
                    n486 = local read "UDPMotorData"() -> (w1118:T5)
                    n487 = local read "Mode"() -> (w1124:T9)
                    n488 = local read "MotorData"() -> (w1114:T7)
                    n489 = local read "RelativePositionRotation"() -> (w1121:dbl)
                    n490 = local read "RelativePositionTranslation"() -> (w1115:dbl)
                    n491 = Not Equal?(x=w1124, y=w1123) -> (x != y?=w1122:bool)
                    n492 = Build Array(w1121, w1115) -> (w1120:dbl[])
                    n493 = call "ReceiveMotorData.vi"("Positions"=w1120, "MotorData Input"=w1114, "Override Data"=w1122, "UDP Input"=w1118) -> ("MotorData Output"=w1119:T40, "Valid Data"=w1116:bool, "UDP Output"=w1117:T5)  [unwired: 2 in, 1 out]
                    n494 = case shown="False" w1116 {
                      tunnel: w1119 -> [_ w1125]
                      frame False {
                      }
                      frame True {
                        n495 = local write "MotorData"(w1125) -> ()
                      }
                    }
                    n496 = local write "UDPMotorData"(w1117) -> ()
                  }
                  frame "Safety" {
                    n497 = local read "Mode"() -> (w1126:T9)
                  }
                  frame "Quit" {
                  }
                }
                n498 = local read "UDPMode"() -> (w1105:T5)
                n499 = To Double Precision Float(number=w1103) -> (double precision float=w1104:dbl)
                n500 = call "SendFloat.vi"("Sent Data"=w1104, "UDP Input"=w1105) -> ("UDP Output"=w1106:T5)  [unwired: 4 in, 1 out]
                n501 = local write "UDPMode"(w1106) -> ()
                n502 = local write "Mode"(w1103) -> ()
              }
            }
          }
          frame #2 {
            # "Calibration Check"
            n503 = local read "UDPCalibration"() -> (w1134:T5)
            n504 = local read "Mode"() -> (w1135:T9)
            n505 = call "ReceiveCalibrationData.vi"("UDP Input"=w1134) -> ("CalibrationData"=w1129:cluster{"value":i8, "motor":i8}, "Did Receive"=w1131:bool, "UDP Output"=w1133:T5)  [unwired: 3 in, 1 out]
            n506 = Equal?(x=ModeControl."Calibrate" ("Mode"), y=w1135) -> (x = y?=w1130:bool)
            n507 = local write "UDPCalibration"(w1133) -> ()
            n508 = And(x=w1131, y=w1130) -> (x .and. y?=w1132:bool)
            n509 = case shown="True" w1132 {
              tunnel: w1129 -> [_ w1138]
              frame False {
              }
              frame True {
                n510 = Unbundle(w1138) -> ("value"=w1137:i8, "motor"=w1136:i8)
                n511 = case shown="0, Default" w1137 {
                  selector: w1137 -> [w1144 w1152 w1160]
                  tunnel: w1136 -> [w1139 w1147 w1155]
                  frame 0, Default {
                    n512 = local read "Calibration"() -> (w1142:T8)
                    n513 = local read "UDPCalibration"() -> (w1145:T5)
                    n514 = To Double Precision Float(number=w1144) -> (double precision float=w1143:dbl)
                    n515 = call "SendFloat.vi"("Sent Data"=w1143, "UDP Input"=w1145) -> ("UDP Output"=w1146:T5)  [unwired: 4 in, 1 out]
                    n516 = Bundle(cluster=w1142, "CalibrationMode"=enum16{"Wait", "Calibrate"}."Wait", "CalibratingMotor"=w1139) -> (w1141:T8)
                    n517 = local write "UDPCalibration"(w1146) -> ()
                    n518 = local write "Calibration"(w1141) -> ()
                  }
                  frame 1 {
                    n519 = local read "Calibration"() -> (w1150:T8)
                    n520 = local read "UDPCalibration"() -> (w1153:T5)
                    n521 = To Double Precision Float(number=w1152) -> (double precision float=w1151:dbl)
                    n522 = call "SendFloat.vi"("Sent Data"=w1151, "UDP Input"=w1153) -> ("UDP Output"=w1154:T5)  [unwired: 4 in, 1 out]
                    n523 = Bundle(cluster=w1150, "CalibrationMode"=enum16{"Wait", "Calibrate"}."Calibrate", "CalibratingMotor"=w1147) -> (w1149:T8)
                    n524 = local write "UDPCalibration"(w1154) -> ()
                    n525 = local write "Calibration"(w1149) -> ()
                  }
                  frame 2 {
                    n526 = case shown="1" w1155 {
                      frame 0, Default {
                        n527 = local read "AbsolutePositionRotation"() -> (w1163:dbl)
                        n528 = Negate(x=w1163) -> (-x=w1164:dbl)
                        n529 = local write "CalibratorRotation"(w1164) -> ()
                      }
                      frame 1 {
                        n530 = local read "AbsolutePositionTranslation"() -> (w1165:dbl)
                        n531 = Negate(x=w1165) -> (-x=w1166:dbl)
                        n532 = local write "CalibratorTranslation"(w1166) -> ()
                      }
                    }
                    n533 = local read "Calibration"() -> (w1158:T8)
                    n534 = local read "UDPCalibration"() -> (w1161:T5)
                    n535 = To Double Precision Float(number=w1160) -> (double precision float=w1159:dbl)
                    n536 = call "SendFloat.vi"("Sent Data"=w1159, "UDP Input"=w1161) -> ("UDP Output"=w1162:T5)  [unwired: 4 in, 1 out]
                    n537 = Bundle(cluster=w1158, "CalibrationMode"=enum16{"Wait", "Calibrate"}."Wait", "CalibratingMotor"=w1155) -> (w1157:T8)
                    n538 = local write "UDPCalibration"(w1162) -> ()
                    n539 = local write "Calibration"(w1157) -> ()
                  }
                }
              }
            }
          }
          frame #3 {
            # "Send Motor Values"
            n540 = local read "RelativePositionRotation"() -> (w1169:dbl)
            n541 = local read "AppliedTorqueRotation [Nmm]"() -> (w1167:dbl)
            n542 = local read "AppliedForceTranslation [N]"() -> (w1170:dbl)
            n543 = local read "VelocityRotation"() -> (w1168:dbl)
            n544 = local read "MotorValues"() -> (w1177:T10)
            n545 = local read "RelativePositionTranslation"() -> (w1172:dbl)
            n546 = local read "VelocityTranslation"() -> (w1171:dbl)
            n547 = Bundle(cluster=w1177, "positionLinear"=w1172, "velocityLinear"=w1171, "appliedForceLinear"=w1170, "positionRotatory"=w1169, "velocityRotatory"=w1168, "appliedTorqueRotatory"=w1167) -> (w1175:T10)
            n548 = local write "MotorValues"(w1175) -> ()
            n549 = Flatten To JSON(anything=w1175) -> (JSON string=w1176:string)  [unwired: 2 in, 1 out]
            n550 = local read "UDPMotorValues"() -> (w1174:T5)
            n551 = call "Send.vi"("SentData"=w1176, "UDP Input"=w1174) -> ("UDP Output"=w1173:T5)  [unwired: 4 in, 1 out]
            n552 = local write "UDPMotorValues"(w1173) -> ()
          }
          frame #4 {
            # "Perturbation sent slower because\notherwise the UDP buffer is overloaded \nand UDP receive in unity becomes slower"
            # "Send Perturbation Values"
            n553 = local read "NewPerturbation"() -> (w1178:bool)
            n554 = case shown="True" w1178 {
              frame False {
              }
              frame True {
                n555 = local read "Perturbation"() -> (w1180:T6)
                n556 = Flatten To JSON(anything=w1180) -> (JSON string=w1183:string)  [unwired: 2 in, 1 out]
                n557 = Concatenate Strings("{\"Items\":" ("string"), w1183, "}" ("string")) -> (w1181:string)
                "JSON string" <- w1181
                n558 = local read "UDPPerturbation"() -> (w1185:T5)
                n559 = local write "NewPerturbation"(FALSE ("NewPerturbation")) -> ()
                n560 = call "Send.vi"("SentData"=w1181, "UDP Input"=w1185) -> ("UDP Output"=w1186:T5)  [unwired: 4 in, 1 out]
                n561 = local write "UDPPerturbation"(w1186) -> ()
              }
            }
          }
          frame #5 {
            # "Game check"
            n562 = local read "UDPGame"() -> (w1189:T5)
            n563 = call "ReceiveGameData.vi"("UDP Input"=w1189) -> ("GameData"=w1187:T46, "Did Receive"=w1188:bool, "UDP Output"=w1190:T5)  [unwired: 3 in, 1 out]
            n564 = local write "UDPGame"(w1190) -> ()
            n565 = case shown="False" w1188 {
              tunnel: w1187 -> [_ w1196]
              frame False {
              }
              frame True {
                n566 = Unbundle(w1196) -> ("gameMode"=w1195:i8, "level"=w1194:dbl, "correctAnswers"=w1193:dbl, "totalAnswers"=w1192:dbl, "repetitions"=w1191:dbl)
                n567 = case shown="0, Default" w1195 {
                  selector: w1195 -> [w1199 w1210 w1221 w1232 w1243]
                  tunnel: w1194 -> [w1204 w1215 w1226 w1237 w1248]
                  tunnel: w1193 -> [w1203 w1214 w1225 w1236 w1247]
                  tunnel: w1192 -> [w1202 w1213 w1224 w1235 w1246]
                  tunnel: w1191 -> [w1201 w1212 w1223 w1234 w1245]
                  frame 0, Default {
                    n568 = local read "Game"() -> (w1207:T4)
                    n569 = local read "UDPGame"() -> (w1198:T5)
                    n570 = To Double Precision Float(number=w1199) -> (double precision float=w1200:dbl)
                    n571 = Bundle(cluster=w1207, "gameMode"=GameMode."NotSave", "level"=w1204, "correctAnswers"=w1203, "totalAnswers"=w1202, "repetitions"=w1201) -> (w1206:T4)
                    n572 = call "SendFloat.vi"("Sent Data"=w1200, "UDP Input"=w1198) -> ("UDP Output"=w1197:T5)  [unwired: 4 in, 1 out]
                    n573 = local write "Game"(w1206) -> ()
                    n574 = local write "UDPGame"(w1197) -> ()
                  }
                  frame 1 {
                    n575 = local read "Game"() -> (w1218:T4)
                    n576 = local read "UDPGame"() -> (w1209:T5)
                    n577 = To Double Precision Float(number=w1210) -> (double precision float=w1211:dbl)
                    n578 = Bundle(cluster=w1218, "gameMode"=GameMode."Calibrate", "level"=w1215, "correctAnswers"=w1214, "totalAnswers"=w1213, "repetitions"=w1212) -> (w1217:T4)
                    n579 = call "SendFloat.vi"("Sent Data"=w1211, "UDP Input"=w1209) -> ("UDP Output"=w1208:T5)  [unwired: 4 in, 1 out]
                    n580 = local write "Game"(w1217) -> ()
                    n581 = local write "UDPGame"(w1208) -> ()
                  }
                  frame 2 {
                    n582 = local read "Game"() -> (w1229:T4)
                    n583 = local read "UDPGame"() -> (w1220:T5)
                    n584 = To Double Precision Float(number=w1221) -> (double precision float=w1222:dbl)
                    n585 = Bundle(cluster=w1229, "gameMode"=GameMode."Training", "level"=w1226, "correctAnswers"=w1225, "totalAnswers"=w1224, "repetitions"=w1223) -> (w1228:T4)
                    n586 = call "SendFloat.vi"("Sent Data"=w1222, "UDP Input"=w1220) -> ("UDP Output"=w1219:T5)  [unwired: 4 in, 1 out]
                    n587 = local write "Game"(w1228) -> ()
                    n588 = local write "UDPGame"(w1219) -> ()
                  }
                  frame 3 {
                    n589 = local read "Game"() -> (w1240:T4)
                    n590 = local read "UDPGame"() -> (w1231:T5)
                    n591 = To Double Precision Float(number=w1232) -> (double precision float=w1233:dbl)
                    n592 = Bundle(cluster=w1240, "gameMode"=GameMode."Test", "level"=w1237, "correctAnswers"=w1236, "totalAnswers"=w1235, "repetitions"=w1234) -> (w1239:T4)
                    n593 = call "SendFloat.vi"("Sent Data"=w1233, "UDP Input"=w1231) -> ("UDP Output"=w1230:T5)  [unwired: 4 in, 1 out]
                    n594 = local write "Game"(w1239) -> ()
                    n595 = local write "UDPGame"(w1230) -> ()
                  }
                  frame 4 {
                    n596 = local read "Game"() -> (w1251:T4)
                    n597 = local read "UDPGame"() -> (w1242:T5)
                    n598 = To Double Precision Float(number=w1243) -> (double precision float=w1244:dbl)
                    n599 = Bundle(cluster=w1251, "gameMode"=GameMode."Summary", "level"=w1248, "correctAnswers"=w1247, "totalAnswers"=w1246, "repetitions"=w1245) -> (w1250:T4)
                    n600 = call "SendFloat.vi"("Sent Data"=w1244, "UDP Input"=w1242) -> ("UDP Output"=w1241:T5)  [unwired: 4 in, 1 out]
                    n601 = local write "Game"(w1250) -> ()
                    n602 = local write "UDPGame"(w1241) -> ()
                  }
                }
              }
            }
          }
          frame #6 {
            # "Safety"
            n603 = local read "Safety Been Triggered"() -> (w1252:bool)
            n604 = case shown="False" w1252 {
              tunnel: [w1256 2] -> w1253
              frame False {
                n605 = local read "SoftSafety"() -> (w1258:bool)
                n606 = Not(x=w1258) -> (.not. x?=w1257:bool)
                n607 = case shown="False" w1257 {
                  tunnel: [0 1] -> w1256
                  frame False {
                  }
                  frame True {
                  }
                }
              }
              frame True {
              }
            }
            n608 = local read "UDPSafety"() -> (w1255:T5)
            n609 = call "SendFloat.vi"("Sent Data"=w1253, "UDP Input"=w1255) -> ("UDP Output"=w1254:T5)  [unwired: 4 in, 1 out]
            n610 = local write "UDPSafety"(w1254) -> ()
          }
          frame #7 {
            n611 = local read "UDPTimestamp"() -> (w1264:T1)
            n612 = call "ReceiveTimeStampData.vi"("UDPTimestamp"=w1264) -> ("TimeStampData"=→"TimeStampData":cluster{"time":string}, "UDP Output"=w1263:T5)  [unwired: 3 in, 2 out]
            n613 = local write "UDPTimestamp"(w1263) -> ()
          }
        }
        n614 = node-c288() -> ()  [unwired: 1 in, 1 out]
      }
      n615 = node-c288(w209) -> ()  [unwired: 1 out]
      n616 = node-c288(w213) -> ()  [unwired: 1 out]
      n617 = node-c288(w211) -> ()  [unwired: 1 out]
    }
    frame #4 {
      # "4: close UDP"
      n618 = local read "UDPPerturbation"() -> (w1269:T5)
      n619 = local read "UDPMotorData"() -> (w1276:T5)
      n620 = local read "UDPConnection"() -> (w1280:T5)
      n621 = local read "UDPMode"() -> (w1277:T5)
      n622 = local read "UDPCalibration"() -> (w1273:T5)
      n623 = local read "UDPGame"() -> (w1270:T5)
      n624 = Unbundle(w1280) -> ("UDP"=w1279:refnum<k16>)  [unwired: 3 out]
      n625 = Unbundle(w1277) -> ("UDP"=w1278:refnum<k16>)  [unwired: 3 out]
      n626 = Unbundle(w1276) -> ("UDP"=w1275:refnum<k16>)  [unwired: 3 out]
      n627 = Unbundle(w1273) -> ("UDP"=w1274:refnum<k16>)  [unwired: 3 out]
      n628 = Unbundle(w1270) -> ("UDP"=w1272:refnum<k16>)  [unwired: 3 out]
      n629 = Unbundle(w1269) -> ("UDP"=w1271:refnum<k16>)  [unwired: 3 out]
      n630 = UDP Close(connection ID=w1279) -> ()  [unwired: 1 in, 2 out]
      n631 = UDP Close(connection ID=w1278) -> ()  [unwired: 1 in, 2 out]
      n632 = UDP Close(connection ID=w1275) -> ()  [unwired: 1 in, 2 out]
      n633 = UDP Close(connection ID=w1274) -> ()  [unwired: 1 in, 2 out]
      n634 = UDP Close(connection ID=w1272) -> ()  [unwired: 1 in, 2 out]
      n635 = UDP Close(connection ID=w1271) -> ()  [unwired: 1 in, 2 out]
    }
  }
